vi "Load Data.vi"(5 "LoadData?":bool, 6 "File Info Buffer Input":T1[](array[typedef])=[{"FilePath"=path "/opticsmac/Documents/Optics2mac/DATA/vclong/01:25:02/visibleperp/v14500aEp02.03T", "Field (T)"=2.0, "Temperature (K)"=4.46, "X-Axis"=enum."cm_1", "Center nm"=689.656101368671, "Current Grating Density"=enum."150", "CCD Parameters"={"Exposure Time (s)"=0.2, "Offset"=0.0, "BkgrdCrct"=FALSE, "Shutter"=FALSE, "Mode"=enum."Regular", "Repetition"=4, "dt or s"=0.0}, "Operation Mode"=enum."NML Data Acquisition", "Exp Index"=0, "Index_repetition"=0, "Index"=0, "Current Detector"=enum."CCD-1024x256"}, {"FilePath"=path "", "Field (T)"=0.0, "Temperature (K)"=0.0, "X-Axis"=enum."Point", "Center nm"=0.0, "Current Grating Density"=enum."150", "CCD Parameters"={"Exposure Time (s)"=0.2, "Offset"=0.0, "BkgrdCrct"=FALSE, "Shutter"=FALSE, "Mode"=enum."Regular", "Repetition"=4, "dt or s"=0.0}, "Operation Mode"=enum."Standby", "Exp Index"=0, "Index_repetition"=0, "Index"=0, "Current Detector"=enum."CCD-1024x256"}, {"FilePath"=path "", "Field (T)"=0.0, "Temperature (K)"=0.0, "X-Axis"=enum."Point", "Center nm"=0.0, "Current Grating Density"=enum."150", "CCD Parameters"={"Exposure Time (s)"=0.2, "Offset"=0.0, "BkgrdCrct"=FALSE, "Shutter"=FALSE, "Mode"=enum."Regular", "Repetition"=4, "dt or s"=0.0}, "Operation Mode"=enum."Standby", "Exp Index"=0, "Index_repetition"=0, "Index"=0, "Current Detector"=enum."CCD-1024x256"}, {"FilePath"=path "", "Field (T)"=0.0, "Temperature (K)"=0.0, "X-Axis"=enum."Point", "Center nm"=0.0, "Current Grating Density"=enum."150", "CCD Parameters"={"Exposure Time (s)"=0.2, "Offset"=0.0, "BkgrdCrct"=FALSE, "Shutter"=FALSE, "Mode"=enum."Regular", "Repetition"=4, "dt or s"=0.0}, "Operation Mode"=enum."Standby", "Exp Index"=0, "Index_repetition"=0, "Index"=0, "Current Detector"=enum."CCD-1024x256"}, {"FilePath"=path "", "Field (T)"=0.0, "Temperature (K)"=0.0, "X-Axis"=enum."Point", "Center nm"=0.0, "Current Grating Density"=enum."150", "CCD Parameters"={"Exposure Time (s)"=0.2, "Offset"=0.0, "BkgrdCrct"=FALSE, "Shutter"=FALSE, "Mode"=enum."Regular", "Repetition"=4, "dt or s"=0.0}, "Operation Mode"=enum."Standby", "Exp Index"=0, "Index_repetition"=0, "Index"=0, "Current Detector"=enum."CCD-1024x256"}, {"FilePath"=path "", "Field (T)"=0.0, "Temperature (K)"=0.0, "X-Axis"=enum."Point", "Center nm"=0.0, "Current Grating Density"=enum."150", "CCD Parameters"={"Exposure Time (s)"=0.2, "Offset"=0.0, "BkgrdCrct"=FALSE, "Shutter"=FALSE, "Mode"=enum."Regular", "Repetition"=4, "dt or s"=0.0}, "Operation Mode"=enum."Standby", "Exp Index"=0, "Index_repetition"=0, "Index"=0, "Current Detector"=enum."CCD-1024x256"}, {"FilePath"=path "", "Field (T)"=0.0, "Temperature (K)"=0.0, "X-Axis"=enum."Point", "Center nm"=0.0, "Current Grating Density"=enum."150", "CCD Parameters"={"Exposure Time (s)"=0.2, "Offset"=0.0, "BkgrdCrct"=FALSE, "Shutter"=FALSE, "Mode"=enum."Regular", "Repetition"=4, "dt or s"=0.0}, "Operation Mode"=enum."Standby", "Exp Index"=0, "Index_repetition"=0, "Index"=0, "Current Detector"=enum."CCD-1024x256"}, {"FilePath"=path "", "Field (T)"=0.0, "Temperature (K)"=0.0, "X-Axis"=enum."Point", "Center nm"=0.0, "Current Grating Density"=enum."150", "CCD Parameters"={"Exposure Time (s)"=0.2, "Offset"=0.0, "BkgrdCrct"=FALSE, "Shutter"=FALSE, "Mode"=enum."Regular", "Repetition"=4, "dt or s"=0.0}, "Operation Mode"=enum."Standby", "Exp Index"=0, "Index_repetition"=0, "Index"=0, "Current Detector"=enum."CCD-1024x256"}, {"FilePath"=path "", "Field (T)"=0.0, "Temperature (K)"=0.0, "X-Axis"=enum."Point", "Center nm"=0.0, "Current Grating Density"=enum."150", "CCD Parameters"={"Exposure Time (s)"=0.2, "Offset"=0.0, "BkgrdCrct"=FALSE, "Shutter"=FALSE, "Mode"=enum."Regular", "Repetition"=4, "dt or s"=0.0}, "Operation Mode"=enum."Standby", "Exp Index"=0, "Index_repetition"=0, "Index"=0, "Current Detector"=enum."CCD-1024x256"}, {"FilePath"=path "", "Field (T)"=0.0, "Temperature (K)"=0.0, "X-Axis"=enum."Point", "Center nm"=0.0, "Current Grating Density"=enum."150", "CCD Parameters"={"Exposure Time (s)"=0.2, "Offset"=0.0, "BkgrdCrct"=FALSE, "Shutter"=FALSE, "Mode"=enum."Regular", "Repetition"=4, "dt or s"=0.0}, "Operation Mode"=enum."Standby", "Exp Index"=0, "Index_repetition"=0, "Index"=0, "Current Detector"=enum."CCD-1024x256"}] {"CCD Parameters"."dt or s" format="%#.6f"; "CCD Parameters"."Repetition" min=1; "CCD Parameters"."Offset" format="%#.2f"; "CCD Parameters"."Exposure Time (s)" min=0.02 max=6000.0 format="%#.2f"; "Center nm" format="%.2f"; "Temperature (K)" format="%.2f"; "Field (T)" format="%.2f"}, 7 "Y-Array in":dbl[](array[numeric]), 8 "Y Array Buffer Input":dbl[][](array[numeric])=array1024x10[10240 elements] format="%.2f", 9 "X-Axis Array Input":dbl[][](array[numeric])=array1024x11[11264 elements] format="%.2f") -> (0 "File Info Buffer Out":T1[](array[typedef])=[{"FilePath"=path "/opticsmac/Documents/Optics2mac/DATA/vclong/01:25:02/visibleperp/v14500aEp02.03T", "Field (T)"=2.0, "Temperature (K)"=4.46, "X-Axis"=enum."cm_1", "Center nm"=689.656101368671, "Current Grating Density"=enum."150", "CCD Parameters"={"Exposure Time (s)"=0.2, "Offset"=0.0, "BkgrdCrct"=FALSE, "Shutter"=FALSE, "Mode"=enum."Regular", "Repetition"=4, "dt or s"=0.0}, "Operation Mode"=enum."NML Data Acquisition", "Exp Index"=0, "Index_repetition"=0, "Index"=0, "Current Detector"=enum."CCD-1024x256"}] {"CCD Parameters"."dt or s" format="%#.6f"; "CCD Parameters"."Repetition" min=1; "CCD Parameters"."Offset" format="%#.2f"; "CCD Parameters"."Exposure Time (s)" min=0.02 max=6000.0 format="%#.2f"; "Center nm" format="%.2f"; "Temperature (K)" format="%.2f"; "Field (T)" format="%.2f"}, 1 "Y-Array out":dbl[](array[numeric]), 2 "Data Array output":dbl[][](array[numeric])=[[156320.0], [157260.0], [158740.0], [160150.0], [162530.0], [164140.0], [166060.0], [167590.0], [169200.0], [171260.0], [172690.0], [174810.0], [176260.0], [178620.0], [180480.0], [181740.0], [183460.0], [185700.0], [187270.0], [189260.0], [191040.0], [192940.0], [193980.0], [196750.0], [198840.0], [200170.0], [202190.0], [203860.0], [205040.0], [206430.0], [209340.0], [210440.0], [213240.0], [214740.0], [216720.0], [218710.0], [220610.0], [222540.0], [224090.0], [226040.0], [227760.0], [228770.0], [231810.0], [233660.0], [235500.0], [237390.0], [239590.0], [241700.0], [243190.0], [245260.0], [245670.0], [248540.0], [250180.0], [252160.0], [254040.0], [255810.0], [257360.0], [258980.0], [260540.0], [261970.0], [262240.0], [265810.0], [266800.0], [268760.0], [270660.0], [271180.0], [273130.0], [274420.0], [276410.0], [276090.0], [278520.0], [280230.0], [281030.0], [281870.0], [283440.0], [285750.0], [286320.0], [287530.0], [288750.0], [288670.0], [290950.0], [292320.0], [293710.0], [294870.0], [295370.0], [296240.0], [297700.0], [298710.0], [298800.0], [301150.0], [302130.0], [303180.0], [303690.0], [304680.0], [305540.0], [306660.0], [307720.0], [308220.0], [307800.0], [310510.0], [310980.0], [311540.0], [312460.0], [312990.0], [313790.0], [314260.0], [315080.0], [314160.0], [316990.0], [317280.0], [317390.0], [317810.0], [318990.0], [319270.0], [319920.0], [320880.0], [320580.0], [321670.0], [323440.0], [324260.0], [324090.0], [325340.0], [326440.0], [327880.0], [328190.0], [329450.0], [328800.0], [331840.0], [332880.0], [333390.0], [334690.0], [335400.0], [336540.0], [337530.0], [338800.0], [338680.0], [340000.0], [341080.0], [341600.0], [342840.0], [343390.0], [344390.0], [345420.0], [346090.0], [346340.0], [346460.0], [349550.0], [349420.0], [350670.0], [351070.0], [351930.0], [353120.0], [353520.0], [354520.0], [354640.0], [355380.0], [356380.0], [357290.0], [358190.0], [358930.0], [359670.0], [359540.0], [360830.0], [361900.0], [360600.0], [362480.0], [363660.0], [364070.0], [364740.0], [364990.0], [366060.0], [366930.0], [367780.0], [367940.0], [368640.0], [369950.0], [370430.0], [371320.0], [371730.0], [372740.0], [373400.0], [373890.0], [374850.0], [374640.0], [376240.0], [378000.0], [377860.0], [379380.0], [380050.0], [380630.0], [381640.0], [382180.0], [382230.0], [383250.0], [385270.0], [385380.0], [387220.0], [387590.0], [387980.0], [389810.0], [390380.0], [391030.0], [390020.0], [392370.0], [393610.0], [394220.0], [394720.0], [395770.0], [397090.0], [397800.0], [398480.0], [398130.0], [399860.0], [400870.0], [401860.0], [402070.0], [403020.0], [404320.0], [405070.0], [406210.0], [407160.0], [406140.0], [408920.0], [410760.0], [410970.0], [412260.0], [413420.0], [414890.0], [415800.0], [416960.0], [417480.0], [417970.0], [420910.0], [421760.0], [422450.0], [425020.0], [425520.0], [427330.0], [429060.0], [430200.0], [429790.0], [433380.0], [434550.0], [435800.0], [437460.0], [439590.0], [441200.0], [442140.0], [444010.0], [444080.0], [447490.0], [449670.0], [449930.0], [451710.0], [453330.0], [454340.0], [456010.0], [459020.0], [459170.0], [459650.0], [463490.0], [464920.0], [466220.0], [467140.0], [469790.0], [470470.0], [471550.0], [473460.0], [473170.0], [476510.0], [478130.0], [479950.0], [481700.0], [482610.0], [484720.0], [486310.0], [487360.0], [488710.0], [488480.0], [491530.0], [493680.0], [494030.0], [496330.0], [496710.0], [499040.0], [500660.0], [502060.0], [501750.0], [505120.0], [507080.0], [509080.0], [510410.0], [511400.0], [513950.0], [515830.0], [516880.0], [518020.0], [517880.0], [521810.0], [522630.0], [524040.0], [526020.0], [526400.0], [527650.0], [529510.0], [531110.0], [530100.0], [534120.0], [534870.0], [536820.0], [537820.0], [538610.0], [539780.0], [542010.0], [541950.0], [543990.0], [542980.0], [545900.0], [546330.0], [547660.0], [548080.0], [549810.0], [550340.0], [551570.0], [553330.0], [551440.0], [554700.0], [555680.0], [557650.0], [558440.0], [559220.0], [559960.0], [561330.0], [562400.0], [562300.0], [561740.0], [564550.0], [565120.0], [566410.0], [566540.0], [567600.0], [569260.0], [569370.0], [570620.0], [569700.0], [573110.0], [574280.0], [574450.0], [575220.0], [576960.0], [577570.0], [580100.0], [580380.0], [581520.0], [581380.0], [585270.0], [586540.0], [587260.0], [589060.0], [590240.0], [591500.0], [593040.0], [594340.0], [593420.0], [596370.0], [597700.0], [598570.0], [601150.0], [601800.0], [604910.0], [606790.0], [607480.0], [608140.0], [609520.0], [612450.0], [613670.0], [614660.0], [615130.0], [616330.0], [617050.0], [618050.0], [620390.0], [620190.0], [624180.0], [625540.0], [626790.0], [628820.0], [629000.0], [630620.0], [631500.0], [632660.0], [632820.0], [635130.0], [637650.0], [638560.0], [639160.0], [640430.0], [641030.0], [642840.0], [644020.0], [644840.0], [643680.0], [646820.0], [648710.0], [649660.0], [649440.0], [650920.0], [652720.0], [653450.0], [654620.0], [654780.0], [656430.0], [657460.0], [657570.0], [659320.0], [659400.0], [660680.0], [661770.0], [662130.0], [662360.0], [661080.0], [664420.0], [664320.0], [665300.0], [665760.0], [665580.0], [666220.0], [667220.0], [667340.0], [666260.0], [666190.0], [667200.0], [666770.0], [667620.0], [667530.0], [667110.0], [667250.0], [666860.0], [666590.0], [664350.0], [667200.0], [666880.0], [666520.0], [666110.0], [665080.0], [664700.0], [665990.0], [664640.0], [663420.0], [662240.0], [662810.0], [663050.0], [662600.0], [662030.0], [662160.0], [660780.0], [660130.0], [657870.0], [655800.0], [658220.0], [657800.0], [655630.0], [654120.0], [654570.0], [652660.0], [652060.0], [651740.0], [649510.0], [647850.0], [647320.0], [646010.0], [644610.0], [642420.0], [640220.0], [640340.0], [638990.0], [637100.0], [633820.0], [634320.0], [632920.0], [631980.0], [630800.0], [629090.0], [628850.0], [627160.0], [625590.0], [623130.0], [621440.0], [621550.0], [620700.0], [618500.0], [617880.0], [616220.0], [615470.0], [612630.0], [611170.0], [607430.0], [608600.0], [606890.0], [604420.0], [603270.0], [601590.0], [599460.0], [597450.0], [596090.0], [592650.0], [591760.0], [591090.0], [589220.0], [586320.0], [586060.0], [584040.0], [581410.0], [580850.0], [578450.0], [574310.0], [574760.0], [572940.0], [570980.0], [569590.0], [567810.0], [565600.0], [563760.0], [561900.0], [557600.0], [557220.0], [554640.0], [552400.0], [551480.0], [549700.0], [548050.0], [546890.0], [545140.0], [542510.0], [538000.0], [538080.0], [536770.0], [534010.0], [531830.0], [530640.0], [529320.0], [527240.0], [525000.0], [520960.0], [521070.0], [520170.0], [518210.0], [516210.0], [515020.0], [512950.0], [511720.0], [510620.0], [508390.0], [503950.0], [504510.0], [503570.0], [501270.0], [500230.0], [498290.0], [497320.0], [496810.0], [493930.0], [490820.0], [491560.0], [489960.0], [489310.0], [486820.0], [485200.0], [484360.0], [481680.0], [480350.0], [478600.0], [474800.0], [474770.0], [472460.0], [471520.0], [469300.0], [467320.0], [465240.0], [463430.0], [461630.0], [456970.0], [457570.0], [455660.0], [453120.0], [450930.0], [448980.0], [446190.0], [444850.0], [443350.0], [441040.0], [436880.0], [436140.0], [434420.0], [432330.0], [430310.0], [428480.0], [426040.0], [424900.0], [422610.0], [419380.0], [418430.0], [416630.0], [416290.0], [414300.0], [412500.0], [411400.0], [410060.0], [408660.0], [407070.0], [403290.0], [403090.0], [401900.0], [400240.0], [399050.0], [397450.0], [395580.0], [394440.0], [393710.0], [390260.0], [390640.0], [388280.0], [386530.0], [385640.0], [384440.0], [382570.0], [381800.0], [381000.0], [378720.0], [377390.0], [376850.0], [375200.0], [374320.0], [373100.0], [371220.0], [370010.0], [368870.0], [367560.0], [364680.0], [364510.0], [363130.0], [361300.0], [360060.0], [358740.0], [357360.0], [355990.0], [354730.0], [352870.0], [351670.0], [351570.0], [350560.0], [349430.0], [349280.0], [348110.0], [348810.0], [348240.0], [347840.0], [346100.0], [347600.0], [347650.0], [348340.0], [348530.0], [348790.0], [348900.0], [348490.0], [349230.0], [348620.0], [347720.0], [349040.0], [348820.0], [348160.0], [348370.0], [348810.0], [348410.0], [348440.0], [348090.0], [346440.0], [347530.0], [347510.0], [347190.0], [346980.0], [346970.0], [347380.0], [346650.0], [346660.0], [346160.0], [345540.0], [346110.0], [346250.0], [346100.0], [346130.0], [345360.0], [345870.0], [346100.0], [345550.0], [344440.0], [345530.0], [345280.0], [345730.0], [345620.0], [345010.0], [345010.0], [345170.0], [345320.0], [343740.0], [344220.0], [345060.0], [344330.0], [345130.0], [344780.0], [344760.0], [344580.0], [344900.0], [344560.0], [343020.0], [343620.0], [343590.0], [343780.0], [342910.0], [343500.0], [343130.0], [343920.0], [343120.0], [342650.0], [342610.0], [343040.0], [343040.0], [342780.0], [342740.0], [342160.0], [341750.0], [341210.0], [340920.0], [339020.0], [340380.0], [339050.0], [338350.0], [337570.0], [337100.0], [336350.0], [335800.0], [335510.0], [333940.0], [333380.0], [334120.0], [334050.0], [333630.0], [334510.0], [334900.0], [335700.0], [337260.0], [338810.0], [339090.0], [343020.0], [345650.0], [347530.0], [350990.0], [354050.0], [357380.0], [360650.0], [363900.0], [365580.0], [369540.0], [373470.0], [375250.0], [377750.0], [379810.0], [381750.0], [383410.0], [384500.0], [386600.0], [385600.0], [387930.0], [389910.0], [390520.0], [391700.0], [392050.0], [391960.0], [391730.0], [392450.0], [390690.0], [393050.0], [392850.0], [393580.0], [394080.0], [392820.0], [393180.0], [392870.0], [392970.0], [393260.0], [390860.0], [391510.0], [391330.0], [390430.0], [389300.0], [388920.0], [388670.0], [388150.0], [388100.0], [386960.0], [388040.0], [388650.0], [387730.0], [387970.0], [386880.0], [387000.0], [386420.0], [386990.0], [385910.0], [383510.0], [384780.0], [384030.0], [384080.0], [383180.0], [381830.0], [381580.0], [381410.0], [381920.0], [379820.0], [381400.0], [381260.0], [381480.0], [381220.0], [381160.0], [380220.0], [379490.0], [379530.0], [379140.0], [377530.0], [378270.0], [377830.0], [377610.0], [376940.0], [376510.0], [376080.0], [375890.0], [376230.0], [373670.0], [374800.0], [374290.0], [373960.0], [373110.0], [373330.0], [372760.0], [371680.0], [371860.0], [371300.0], [367850.0], [368940.0], [368290.0], [367740.0], [367630.0], [366490.0], [366590.0], [365400.0], [364700.0], [362360.0], [362780.0], [362460.0], [361600.0], [361410.0], [360710.0], [359930.0], [359220.0], [358090.0], [358030.0], [355680.0], [356970.0], [355700.0], [355970.0], [355130.0], [354980.0], [354470.0], [354120.0], [353610.0], [351920.0], [353430.0], [353730.0], [353240.0], [352810.0], [352730.0], [352930.0], [353230.0], [352990.0], [352320.0], [352370.0], [353100.0], [353530.0], [354110.0], [353310.0], [354720.0], [354820.0], [355090.0], [356000.0], [354730.0], [356760.0], [357560.0], [358070.0], [358370.0], [359300.0], [359980.0], [361140.0], [362240.0], [362300.0], [362850.0], [364220.0], [365530.0], [366740.0], [367400.0], [368790.0], [369320.0], [370690.0], [372240.0], [370660.0], [374080.0], [374970.0], [376000.0], [377270.0], [378520.0], [379880.0], [381660.0], [383190.0], [384070.0], [384140.0], [386260.0], [388280.0], [389600.0], [391170.0], [392920.0], [393800.0], [395680.0], [397070.0], [397120.0], [400470.0], [401730.0], [403790.0], [406060.0], [406910.0], [408630.0], [411080.0], [413560.0], [413080.0], [415620.0], [418270.0], [419420.0], [421620.0], [423980.0], [426180.0], [427900.0], [429930.0], [431090.0], [432040.0], [435340.0], [437000.0], [439230.0], [441180.0], [442820.0], [445160.0], [447410.0], [448810.0], [450420.0], [452100.0], [453960.0], [456590.0], [457360.0], [460200.0], [462210.0], [464290.0], [466050.0], [467300.0], [467040.0], [470870.0], [472490.0], [475020.0], [476600.0], [479850.0], [481770.0], [483830.0], [485770.0], [487240.0], [489490.0], [491690.0], [493030.0], [495820.0], [497760.0], [499750.0], [502150.0], [504600.0], [507830.0], [505690.0], [510100.0], [512330.0], [514740.0], [516420.0], [517990.0], [520020.0], [521630.0], [523580.0], [524160.0], [525290.0], [528610.0], [529240.0], [531820.0], [533720.0], [536570.0], [537640.0], [539530.0], [541010.0], [542030.0], [545080.0], [547040.0], [548830.0], [550910.0], [551940.0], [553730.0], [556100.0], [556780.0], [557540.0], [560360.0], [562490.0], [563420.0], [565890.0], [565840.0], [556840.0]] format="%.2f", 3 "X-Axis Array output":dbl[][](array[numeric])=[[569.9785612360697], [570.2125422703458], [570.4467790424538], [570.6811447284165], [570.9150664597546], [571.149498604365], [571.3834857004028], [571.6176645935107], [571.8520993896819], [572.0859594909508], [572.3203947937624], [572.5543820427264], [572.7885606964572], [573.0228668580249], [573.257108052247], [573.4911554110627], [573.7251368031901], [573.959566566362], [574.1935440459157], [574.4277123674399], [574.6618137673706], [574.8960415039011], [575.1301372348125], [575.3644236893715], [575.598512842311], [575.8325335034439], [576.0667445331885], [576.3007569575373], [576.5350245027386], [576.7690927467231], [577.0034161532332], [577.237539561065], [577.4715925143892], [577.7057701635956], [577.9398116322578], [578.1740428085933], [578.4081372083515], [578.6424212478402], [578.8765679131884], [579.1105766403081], [579.3447090835253], [579.5787684902041], [579.8130170966701], [580.047060849429], [580.281030556443], [580.5151232693252], [580.7494049303583], [580.9836120636254], [581.2176123012891], [581.4518011094145], [581.6858482876963], [581.9197532660246], [582.1541773939755], [582.3881280180103], [582.6222667533773], [582.8561957158248], [583.0903790087464], [583.3244182677612], [583.5585789664744], [583.7926614753968], [584.0268652358009], [584.2609236252295], [584.4949027934747], [584.7290026613164], [584.9632901260253], [585.1970965537491], [585.4314246553758], [585.6652705642005], [585.8996385960471], [586.1334561771368], [586.3675276076606], [586.6017860649538], [586.8358954680223], [587.0697879210392], [587.3038668912492], [587.5378629136461], [587.771977993909], [588.0059420756725], [588.2401600748535], [588.4741589158375], [588.708343997923], [588.9423768195961], [589.1762567952333], [589.4103226008467], [589.644574458002], [589.8786048264974], [590.1125489853926], [590.3466787810725], [590.580585701375], [590.8147462283345], [591.0486831331444], [591.2828053689865], [591.5168398027985], [591.7509911829102], [591.9849857807982], [592.2188230044163], [592.4528450349327], [592.6870520915197], [592.9211010776456], [593.1549913992526], [593.3890663196886], [593.6229131024171], [593.8570131497573], [594.0912979084737], [594.3250087204426], [594.5593177431829], [594.7930515160485], [595.0273840434575], [595.2611400157674], [595.4950797219038], [595.7292033785758], [595.9631643548844], [596.1973091705743], [596.4312906493552], [596.6651081898347], [596.8991091280797], [597.1332936799505], [597.367313577354], [597.6010984655192], [597.8351362188375], [598.0692874950604], [598.3033425992447], [598.5371611499348], [598.7712325507011], [599.0050666235196], [599.2390834029617], [599.4732831032484], [599.7069634997492], [599.9411776423483], [600.1752230319117], [600.4090990591753], [600.6431574309179], [600.877045769227], [601.1111163290896], [601.3449455547924], [601.5790274511555], [601.8128672292677], [602.0469596628537], [602.2808091924991], [602.514911361466], [602.748769839205], [602.9828099258036], [603.216747558975], [603.450795659303], [603.6846695575144], [603.918368637198], [604.1526051721127], [604.386238691957], [604.6204813770987], [604.8541911551888], [605.0880816793274], [605.3220815938698], [605.5559760805389], [605.7900513892174], [606.0238773407672], [606.2578838686974], [606.4917838131607], [606.7257924111401], [606.9596218926068], [607.1936316772918], [607.4275337172702], [607.661543913694], [607.89537360751], [608.1293833271114], [608.3631395625441], [608.597147914069], [608.8309743709509], [609.0649805717787], [609.2987316709077], [609.5327348245695], [609.766845166383], [610.0004813285047], [610.234587524326], [610.4685459360591], [610.7023195953143], [610.9362359168458], [611.1700032032709], [611.4039129492185], [611.6380018097078], [611.871904377806], [612.1056200202532], [612.339514274836], [612.5735507012292], [612.8074360352316], [613.0410963234237], [613.2749348664887], [613.5089886256392], [613.7428164669835], [613.976822614781], [614.2106388600395], [614.4445963888058], [614.6784001409918], [614.9123449658256], [615.1461353534156], [615.3800666016712], [615.6138057407791], [615.84772250912], [616.0814464485342], [616.3153478591558], [616.5494269431979], [616.783275246885], [617.0169663999313], [617.2507974982777], [617.4848058938925], [617.718656418489], [617.9522366370846], [618.1860308913114], [618.4200021185717], [618.6537767574555], [618.887728205784], [619.1214449036934], [619.3553381897889], [619.5890333709201], [619.8229424919921], [620.0569907459521], [620.2908400791476], [620.5244522387055], [620.7582780601838], [620.9922801684296], [621.2260441981704], [621.4600220047827], [621.6937609388353], [621.927675763351], [622.1613886642195], [622.3952772840859], [622.6289632400833], [622.8627868559894], [623.0964449244505], [623.3302404222478], [623.564249405239], [623.7980161517389], [624.0315779479429], [624.2656952832338], [624.4992266333307], [624.7333139161664], [624.9668138959906], [625.2008320299667], [625.4346816845912], [625.6682858277579], [625.9020645416273], [626.1360563077307], [626.3698016352901], [626.6033381191387], [626.8374325277452], [627.0708955086782], [627.3049551761817], [627.5383820307816], [627.7724060186698], [628.0061809545841], [628.2397446303601], [628.4734821015171], [628.7073935621099], [628.9410929104458], [629.174966062032], [629.4086263402593], [629.6424215186693], [629.8760417482332], [630.1097966320631], [630.3437250790315], [630.5774389737746], [630.8113651016672], [631.0449981919082], [631.2788433245437], [631.5124723713293], [631.7462744089887], [631.979820588088], [632.2135395073883], [632.4474704201107], [632.6811445201904], [632.9149913579909], [633.1486196432628], [633.3824204709198], [633.6160019721298], [633.8497165843745], [634.083642939327], [634.3173098008219], [634.5507950475294], [634.7848064008625], [635.0182028215893], [635.2521650218868], [635.4859053073872], [635.7194229977089], [635.9531123694371], [636.1869340871817], [636.4205718226408], [636.6543416437656], [636.8879267568933], [637.1216436942005], [637.3555322273472], [637.5891955529648], [637.8226329866419], [638.0566389917908], [638.2899812471152], [638.5239322074651], [638.7576562808872], [638.9911129066096], [639.2247402447219], [639.4585384825399], [639.692148153701], [639.9258885830285], [640.1597998900476], [640.3934417207572], [640.626893454426], [640.8605154571301], [641.0942677783141], [641.3277890211948], [641.5615206436516], [641.7953824702491], [642.0290123129754], [642.2628123120527], [642.496379526627], [642.7301166825058], [642.9635798805645], [643.1972531457308], [643.4310963211325], [643.6646645385084], [643.8984023899698], [644.1319453967337], [644.3656173302636], [644.5990530940628], [644.8326174473822], [645.066391757513], [645.2999289791973], [645.5336353598614], [645.7674703591786], [646.0011080433068], [646.2344662336811], [646.4684012053606], [646.7016887629393], [646.9355534678967], [647.1691783656399], [647.4025627531603], [647.6361155291756], [647.8697958862166], [648.103685956802], [648.3372934247961], [648.5706996532427], [648.8042328900535], [649.0379343657853], [649.2713925888587], [649.5050188216914], [649.7388132457125], [649.9723634797793], [650.2060403887166], [650.4395135398449], [650.6731130749776], [650.9069218357406], [651.140443235878], [651.3737179101438], [651.6075744289843], [651.8411839880306], [652.074545875291], [652.308074911467], [652.5417296931276], [652.7755935365271], [653.0087505723392], [653.242532621299], [653.476023396739], [653.7097228787869], [653.9431301933079], [654.1767042437094], [654.4104452087186], [654.643892901282], [654.8775490900751], [655.1109530200998], [655.3444814426795], [655.5782183880856], [655.8116601135669], [656.0453101793759], [656.2786641242704], [656.5121841352549], [656.7458703896632], [656.9793015591454], [657.2128987273431], [657.4466198608332], [657.6801271223752], [657.913335337913], [658.147174305523], [658.3807139200136], [658.613995727499], [658.8474853001089], [659.0810980625783], [659.3148765516596], [659.5483961348145], [659.7816135745428], [660.0154639560657], [660.2486287429053], [660.4823417401426], [660.7158365714216], [660.9494538905137], [661.182809556881], [661.4163300591503], [661.6500155720365], [661.883438448266], [662.1170260806862], [662.3503502177476], [662.5838388554693], [662.8174492648519], [663.0508380632363], [663.2843483160027], [663.5175931625031], [663.7514753723896], [663.9846183813248], [664.2183560764337], [664.4518272425249], [664.6850311438042], [664.9188305532281], [665.1523192315412], [665.3855828228633], [665.6189668124593], [665.852557875202], [666.085836348174], [666.3192783345766], [666.5529273943554], [666.7862627704383], [667.0197615677935], [667.2534239581643], [667.4867715072842], [667.7203258631687], [667.9536080127298], [668.1870096223497], [668.4206180344975], [668.6539095684766], [668.8873640056947], [669.1209815168397], [669.3543684916073], [669.5878745482652], [669.8210616205942], [670.0544550114707], [670.2880111068818], [670.5217300770249], [670.7551287876049], [670.9882943339953], [671.2215780432409], [671.4550240212379], [671.6886764964981], [671.9220066530777], [672.1554989737157], [672.3887121169042], [672.62204296728], [672.8555800261507], [673.0892793113455], [673.3226982539178], [673.555791797064], [673.7895344693354], [674.0225077441829], [674.2560861488573], [674.4893822263485], [674.7228398030073], [674.9565035354801], [675.1897949282433], [675.4228466922716], [675.6565052063161], [675.8898793213142], [676.1233700656283], [676.3566201244364], [676.5899864682003], [676.8235139064099], [677.0567997098706], [677.2902015884175], [677.5233161643367], [677.7570398537687], [677.9899821683338], [678.2235787871269], [678.4568869138255], [678.6903556112117], [678.923489897466], [679.1568294491952], [679.3902843739306], [679.6239449568319], [679.8572698087271], [680.0903032405772], [680.3239484726362], [680.5573019943785], [680.7903630401039], [681.0235384746044], [681.2569190155838], [681.4904595661528], [681.7236610504576], [681.9570676059204], [682.1905885945728], [682.4238147784475], [682.6572459966719], [682.8903360147227], [683.1235852620623], [683.3569939019063], [683.5905620976938], [683.8237876919464], [684.0572181797826], [684.2903508110712], [684.5235966447381], [684.7570473302867], [684.9901532665468], [685.2234179653401], [685.4568874728135], [685.6900110634476], [685.9232932784943], [686.1567342799079], [686.3898281317407], [686.623126445873], [686.856583406323], [687.0897381470143], [687.3230050969968], [687.5564766544361], [687.789598713726], [688.0228789107953], [688.2563636660593], [688.4894977448944], [688.7227898169376], [688.9562400428498], [689.1893847335801], [689.4226872713384], [689.656101368671], [689.8892552578118], [690.1225668461884], [690.3555243307512], [690.5891514513938], [690.8224240958862], [691.055388021864], [691.2885091242657], [691.5217875622108], [691.7552234950339], [691.9883494570898], [692.2216326020165], [692.4550730888359], [692.6882025052314], [692.9214420615496], [693.154885662274], [693.3879701385429], [693.621258407787], [693.854186542698], [694.0877416377679], [694.3210303127407], [694.5539105419989], [694.7875127414463], [695.0202343195562], [695.2536311046698], [695.4867123324328], [695.7199498918577], [695.9532966403738], [696.1863739873769], [696.4195601403177], [696.6529499510642], [696.8859745504592], [697.119155091584], [697.352491731027], [697.5855094050058], [697.8191583932959], [698.052012237179], [698.2854977081029], [698.5186629315928], [698.7514594284022], [698.9849359872462], [699.2180434308635], [699.4513541829035], [699.6842947933923], [699.9173906095419], [700.1506896586855], [700.3840963837952], [700.6171794206019], [700.8504176459352], [701.0833312166185], [701.316351615363], [701.5495750281236], [701.7829536098167], [702.0159581115853], [702.2491655476285], [702.4824797851062], [702.7155150939038], [702.9486568085897], [703.1819532746579], [703.4149214500542], [703.6480440439698], [703.8813212099857], [704.1142689444213], [704.347370916823], [704.5806272804261], [704.8140381886692], [705.0470698099189], [705.2803041521312], [705.5131581648886], [705.7461659857089], [705.9793764395791], [706.2126923662339], [706.4456751899384], [706.6788117885895], [706.9121023144813], [707.145058585656], [707.3781684445645], [707.6114320431471], [707.844311302739], [708.0773928590395], [708.3106279657914], [708.5434774801842], [708.7764801384772], [709.0096851830824], [709.2429946150864], [709.4759660859403], [709.7090906595838], [709.9423684869894], [710.1753071906984], [710.4083988032949], [710.6416434753902], [710.8745478587958], [711.1075555733332], [711.3407655013067], [711.5735845262209], [711.806605481884], [712.039729591787], [712.273055997113], [712.5059900253336], [712.7390764558131], [712.9723154381692], [713.2052103819556], [713.4382575273833], [713.6714570237015], [713.9042615343643], [714.1372677833431], [714.3704261805599], [714.6031883165729], [714.8366510991905], [715.0697172024965], [715.3024856342254], [715.5353556570582], [715.7683773530886], [716.0015508705467], [716.2348763578561], [716.4678526681815], [716.70047897149], [716.9337583312919], [717.1666873272304], [717.3997174678144], [717.6329493880252], [717.8658297547535], [718.0988109574024], [718.3319938265538], [718.5647735268387], [718.7977041432862], [719.0307858227071], [719.2640692336621], [719.4969479698311], [719.7299775548271], [719.9626013176862], [720.1959326794039], [720.4289084763316], [720.6620350524665], [720.8947542938646], [721.1276746688834], [721.3606947886973], [721.5939163995395], [721.8267291591917], [722.0597431103231], [722.2928566012382], [722.5256108516573], [722.758515157566], [722.991569664121], [723.2242637220327], [723.457618736422], [723.6906129341463], [723.9231942941278], [724.1564885199274], [724.3893694728172], [724.6224515350356], [724.8551192291109], [725.0879877278858], [725.3209545223762], [725.5540710668876], [725.7868230850675], [726.0197244811866], [726.2528269072134], [726.48602752403], [726.7188106338266], [726.9517945770532], [727.1844115522902], [727.4176941796782], [727.6505577576538], [727.8831048166599], [728.1162665155825], [728.349111385633], [728.5820533875615], [728.8151444370693], [729.0479175287326], [729.2807874181402], [729.5138061200224], [729.7464537279817], [729.979249769529], [730.2121423154941], [730.4452356174513], [730.677956402216], [730.9108255245195], [731.1437909220073], [731.3769571118838], [731.6096970864359], [731.8426375379956], [732.0756740332973], [732.3083352779314], [732.5411444538945], [732.7741541396158], [733.00725963518], [733.2399884457418], [733.4728650854023], [733.705837124326], [733.9384837705344], [734.1712780007656], [734.4041672846467], [734.6372570710988], [734.8699674863099], [735.1027726080894], [735.335725280871], [735.5683501029508], [735.8010692827844], [736.0339357646509], [736.266949688449], [736.4995814754819], [736.7323603142135], [736.9652863441196], [737.1983597048528], [737.4310494767265], [737.6638861876831], [737.8968168039282], [738.1294157114595], [738.3626404655607], [738.5950004475568], [738.827986486663], [739.0605861515492], [739.2939194374667], [739.5262785318844], [739.759318149966], [739.9919699308888], [740.2247680942306], [740.4577127781887], [740.6902683570029], [740.923506160012], [741.1563544603426], [741.3887587074263], [741.6218995732415], [741.8545959196258], [742.0874921153204], [742.319942649985], [742.5525927014187], [742.7858735473785], [743.0182227395939], [743.251256813197], [743.4838972932176], [743.7166834535531], [743.949669480017], [744.1821525352484], [744.4148350535932], [744.6476631225607], [744.8806368787639], [745.1131600591114], [745.3458827064325], [745.5786964867079], [745.8117100741464], [746.044271461905], [746.2770323186055], [746.5098840387293], [746.7423365567711], [746.9754787791853], [747.2082213919584], [747.4405635117911], [747.6735960821903], [747.9062277508853], [748.1390042269853], [748.3713787120207], [748.6043901407339], [748.8370538614945], [749.0698622494173], [749.3027606099149], [749.5353100668009], [749.7679490163653], [750.0007324225902], [750.233110761735], [750.4662381436045], [750.6989050792552], [750.9317163270375], [751.1641209978687], [751.3966695663436], [751.6293621661489], [751.8621989311368], [752.0951247563495], [752.3276974878573], [752.5604141022473], [752.7932193915123], [753.0256703803677], [753.2582095581994], [753.4909478437834], [753.7237745161723], [753.9561899913641], [754.1887488443199], [754.4214512077558], [754.6543528300939], [754.886786149125], [755.1199195325336], [755.352026869878], [755.5848902206728], [755.8173393207254], [756.0504897014332], [756.282610994813], [756.5154896546507], [756.7478966066582], [756.9810619453718], [757.2131951498128], [757.4460870734576], [757.678505615293], [757.9116278002577], [758.1437708605221], [758.376673992457], [758.6091020646318], [758.8416164156413], [759.0743296109781], [759.3071855819429], [759.5396210802211], [759.7721989261688], [760.0049192505907], [760.2377257429041], [760.470166621687], [760.7026931698258], [760.9354185044483], [761.1682297003532], [761.4006172549887], [761.6332033995022], [761.8658750007254], [762.0981216216317], [762.331077409063], [762.5636077837489], [762.7962800570787], [763.028525791631], [763.2614819049635], [763.494011045611], [763.7266249495914], [763.9588676786684], [764.1918219982317], [764.4242907165299], [764.6569580124176], [764.8891385070066], [765.1220889028531], [765.354551991043], [765.5871563782794], [765.8193294593644], [766.0522164830647], [766.2846717622601], [766.5173255372134], [766.7494316769349], [766.9823103469583], [767.2147556975435], [767.4473419828546], [767.6800693311062], [767.9123044148358], [768.1447376721959], [768.3772540222936], [768.6099688712962], [768.8421897346353], [769.0751863373794], [769.3076884415051], [769.5397528529897], [769.7725938404661], [770.0049388598031], [770.237424181634], [770.4700499330804], [770.7028162414178], [770.935142822511], [771.1676095144611], [771.4001583328958], [771.6323241301861], [771.8652115298873], [772.0975991685474], [772.3301850319092], [772.5622699146975], [772.7951358583659], [773.0275003023413], [773.260062914976], [773.4921228060754], [773.7249066429874], [773.9572456645357], [774.1897242644668], [774.4224011359809], [774.6545146774336], [774.887471053337], [775.1198635062366], [775.3518670192801], [775.5845968899058], [775.8168787295938], [776.0492409306255], [776.2818012103022], [776.5145009153999], [776.7466920565741], [776.9790220975414], [777.2115501529908], [777.4441584030325], [777.6763153210132], [777.9092609869617], [778.1416958032858], [778.3736778954418], [778.6063903663274], [778.8386496550254], [779.07104755156], [779.303584180046], [779.5356068875016], [779.7684209628557], [780.00078000078], [780.2332775588451], [780.4652594258139], [780.698034005651], [780.9302923623035], [781.1627485455421], [781.3952835316442], [781.6273603772329], [781.8602317940714], [782.0925849450691], [782.3244785509395], [782.5571077545219], [782.7892769488586], [783.0215839440813], [783.254028862911], [783.4866118282148], [783.718733143159], [783.9515922141052], [784.1839291152866], [784.4158629723539], [784.6485353086861], [784.8806839560654], [785.1130302081439], [785.3454538315042], [785.578015108261], [785.8101714378415], [786.0424046848741], [786.2747752379038], [786.507283218738], [786.7393242969458], [786.9721676226125], [787.2044831295315], [787.436269760594], [787.6688593962626], [787.9009802365349], [788.1332379261105], [788.3656325860463], [788.5981036063885], [788.8307725349462], [789.0629707696862], [789.2952449046714], [789.5277167020348], [789.7596554673503], [789.9917305455472], [790.2246128574637], [790.4563511392375], [790.6888359137664], [790.921457482874], [791.1536658383246], [791.3859494216275], [791.6183694424177], [791.8502524563984], [792.0829453171151], [792.3151619255425], [792.5475147327539], [792.7793900894214], [793.0119538807791], [793.2441011184819], [793.4763843140877], [793.7087420662068], [793.9406203746562], [794.1733117283034], [794.4054615996114], [794.637808897988], [794.8696134387612], [795.1021706289258], [795.334246207211], [795.5664573021658], [795.7988040325239], [796.0312865171579], [796.263285699578], [796.4954201513341], [796.7276899907661], [796.9600953363514], [797.1926363067062], [797.4246299392921], [797.656820772043], [797.8890846903162], [798.1209240494411], [798.3534583634893], [798.5855677027041], [798.817749730399], [799.0500668072964], [799.2825814392066], [799.5145447623521], [799.746642762781], [799.9788755578173], [800.2112432649212], [800.4431203086334], [800.675757829049], [800.9079041945205], [801.1395584328427], [801.3719738621262], [801.6044614298306], [801.8365188455465], [802.0687106573157], [802.3009741218762], [802.5328060755495], [802.7653384428093], [802.9974388773092], [803.2296105575747], [803.461286112407], [803.6937892129381], [803.9257326499442], [804.1578100018542], [804.3900213846773], [804.6223669145569], [804.8542140995525], [805.0868912041427], [805.3189428710359], [805.5511917162275], [805.7829404892315], [806.0154570780633], [806.2474730952305], [806.4795592085159], [806.7118425298484], [806.9435602081946], [807.1761109293301], [807.408159095993], [807.640277020615], [807.8725284445685], [808.1043395281949], [808.3362198725039], [808.5688717882188]] format="%.2f", 4 "Dataload Type":u8(ring) items=["None", "Buffer", "File"])   [LabVIEW 2020]
doc: "This is a sub VI to load data into PlotBuffer.\nIt uses the x-arrayPlotBuffer (nm), data-arrayPlotBuffer and FileInfoBuffer as input and output. \nIt should be used in a shift-register settings"
uses:
  Globals and TypeDefs/Type Definitions.llb/FileInfoParameter.ctt
  Globals and TypeDefs/Type Definitions.llb/Wavelength Unit.ctt
  Globals and TypeDefs/Type Definitions.llb/McPherson Grating Density.ctl
  Globals and TypeDefs/Type Definitions.llb/CCDParameter.ctt
  Globals and TypeDefs/Type Definitions.llb/OperationMode.ctt
  Globals and TypeDefs/Type Definitions.llb/ListOfDetectors.ctt
  Globals and TypeDefs/Type Definitions.llb/3 way Status.ctl
  File and save/X-Axis Converter.llb/X-Axis Converter.vi
  File and save/X-Axis_Generator_morph.vi
panel:
  out "File Contents":string="#   FILE:   v14500aEp02.03T\r#   Sample:   NENB #3(transmittance)\r#   Friday, January 25, 2002 9:15 PM\r#   Magnet ID: Cell 8\r#   Magnetic Field (Tesla):      2.03\r#   Temperature (K):     -1.00\r#   Exposure Time:      3.00\r#   User Name:   VCLong\r#   Voigt probe\r#   sample axis parallel to field\r#   100 um slit\r#   no filter  in collection\r#   900nm short pass filter in front of source\r#   visible polarizer perpendicular to sample axis\r#   150 line grating\r#   T=4.5K\r#   Unit\r#   cm_1            Response\r17544.52\t 1.5632E+5\r17537.32\t 1.5726E+5\r17530.12\t 1.5874E+5\r17522.92\t 1.6015E+5\r17515.74\t 1.6253E+5\r17508.55\t 1.6414E+5\r17501.38\t 1.6606E+5\r17494.21\t 1.6759E+5\r17487.04\t 1.6920E+5\r17479.89\t 1.7126E+5\r17472.73\t 1.7269E+5\r17465.59\t 1.7481E+5\r17458.45\t 1.7626E+5\r17451.31\t 1.7862E+5\r17444.18\t 1.8048E+5\r17437.06\t 1.8174E+5\r17429.95\t 1.8346E+5\r17422.83\t 1.8570E+5\r17415.73\t 1.8727E+5\r17408.63\t 1.8926E+5\r17401.54\t 1.9104E+5\r17394.45\t 1.9294E+5\r17387.37\t 1.9398E+5\r17380.29\t 1.9675E+5\r17373.22\t 1.9884E+5\r17366.16\t 2.0017E+5\r17359.10\t 2.0219E+5\r17352.05\t 2.0386E+5\r17345.00\t 2.0504E+5\r17337.96\t 2.0643E+5\r17330.92\t 2.0934E+5\r17323.89\t 2.1044E+5\r17316.87\t 2.1324E+5\r17309.85\t 2.1474E+5\r17302.84\t 2.1672E+5\r17295.83\t 2.1871E+5\r17288.83\t 2.2061E+5\r17281.83\t 2.2254E+5\r17274.84\t 2.2409E+5\r17267.86\t 2.2604E+5\r17260.88\t 2.2776E+5\r17253.91\t 2.2877E+5\r17246.94\t 2.3181E+5\r17239.98\t 2.3366E+5\r17233.03\t 2.3550E+5\r17226.08\t 2.3739E+5\r17219.13\t 2.3959E+5\r17212.19\t 2.4170E+5\r17205.26\t 2.4319E+5\r17198.33\t 2.4526E+5\r17191.41\t 2.4567E+5\r17184.50\t 2.4854E+5\r17177.58\t 2.5018E+5\r17170.68\t 2.5216E+5\r17163.78\t 2.5404E+5\r17156.89\t 2.5581E+5\r17150.00\t 2.5736E+5\r17143.12\t 2.5898E+5\r17136.24\t 2.6054E+5\r17129.37\t 2.6197E+5\r17122.50\t 2.6224E+5\r17115.64\t 2.6581E+5\r17108.79\t 2.6680E+5\r17101.94\t 2.6876E+5\r17095.09\t 2.7066E+5\r17088.26\t 2.7118E+5\r17081.42\t 2.7313E+5\r17074.60\t 2.7442E+5\r17067.77\t 2.7641E+5\r17060.96\t 2.7609E+5\r17054.15\t 2.7852E+5\r17047.34\t 2.8023E+5\r17040.54\t 2.8103E+5\r17033.75\t 2.8187E+5\r17026.96\t 2.8344E+5\r17020.18\t 2.8575E+5\r17013.40\t 2.8632E+5\r17006.63\t 2.8753E+5\r16999.86\t 2.8875E+5\r16993.10\t 2.8867E+5\r16986.34\t 2.9095E+5\r16979.59\t 2.9232E+5\r16972.85\t 2.9371E+5\r16966.11\t 2.9487E+5\r16959.37\t 2.9537E+5\r16952.64\t 2.9624E+5\r16945.92\t 2.9770E+5\r16939.20\t 2.9871E+5\r16932.49\t 2.9880E+5\r16925.78\t 3.0115E+5\r16919.08\t 3.0213E+5\r16912.38\t 3.0318E+5\r16905.69\t 3.0369E+5\r16899.00\t 3.0468E+5\r16892.32\t 3.0554E+5\r16885.65\t 3.0666E+5\r16878.98\t 3.0772E+5\r16872.31\t 3.0822E+5\r16865.65\t 3.0780E+5\r16859.00\t 3.1051E+5\r16852.35\t 3.1098E+5\r16845.71\t 3.1154E+5\r16839.07\t 3.1246E+5\r16832.43\t 3.1299E+5\r16825.81\t 3.1379E+5\r16819.18\t 3.1426E+5\r16812.57\t 3.1508E+5\r16805.95\t 3.1416E+5\r16799.35\t 3.1699E+5\r16792.75\t 3.1728E+5\r16786.15\t 3.1739E+5\r16779.56\t 3.1781E+5\r16772.97\t 3.1899E+5\r16766.39\t 3.1927E+5\r16759.82\t 3.1992E+5\r16753.25\t 3.2088E+5\r16746.68\t 3.2058E+5\r16740.12\t 3.2167E+5\r16733.57\t 3.2344E+5\r16727.02\t 3.2426E+5\r16720.47\t 3.2409E+5\r16713.93\t 3.2534E+5\r16707.40\t 3.2644E+5\r16700.87\t 3.2788E+5\r16694.35\t 3.2819E+5\r16687.83\t 3.2945E+5\r16681.31\t 3.2880E+5\r16674.81\t 3.3184E+5\r16668.30\t 3.3288E+5\r16661.80\t 3.3339E+5\r16655.31\t 3.3469E+5\r16648.82\t 3.3540E+5\r16642.34\t 3.3654E+5\r16635.86\t 3.3753E+5\r16629.39\t 3.3880E+5\r16622.92\t 3.3868E+5\r16616.46\t 3.4000E+5\r16610.00\t 3.4108E+5\r16603.55\t 3.4160E+5\r16597.10\t 3.4284E+5\r16590.66\t 3.4339E+5\r16584.22\t 3.4439E+5\r16577.79\t 3.4542E+5\r16571.36\t 3.4609E+5\r16564.94\t 3.4634E+5\r16558.53\t 3.4646E+5\r16552.11\t 3.4955E+5\r16545.71\t 3.4942E+5\r16539.30\t 3.5067E+5\r16532.91\t 3.5107E+5\r16526.52\t 3.5193E+5\r16520.13\t 3.5312E+5\r16513.75\t 3.5352E+5\r16507.37\t 3.5452E+5\r16501.00\t 3.5464E+5\r16494.63\t 3.5538E+5\r16488.27\t 3.5638E+5\r16481.91\t 3.5729E+5\r16475.56\t 3.5819E+5\r16469.21\t 3.5893E+5\r16462.87\t 3.5967E+5\r16456.53\t 3.5954E+5\r16450.20\t 3.6083E+5\r16443.87\t 3.6190E+5\r16437.55\t 3.6060E+5\r16431.23\t 3.6248E+5\r16424.92\t 3.6366E+5\r16418.61\t 3.6407E+5\r16412.31\t 3.6474E+5\r16406.01\t 3.6499E+5\r16399.71\t 3.6606E+5\r16393.43\t 3.6693E+5\r16387.14\t 3.6778E+5\r16380.86\t 3.6794E+5\r16374.59\t 3.6864E+5\r16368.32\t 3.6995E+5\r16362.06\t 3.7043E+5\r16355.80\t 3.7132E+5\r16349.54\t 3.7173E+5\r16343.29\t 3.7274E+5\r16337.05\t 3.7340E+5\r16330.81\t 3.7389E+5\r16324.57\t 3.7485E+5\r16318.34\t 3.7464E+5\r16312.12\t 3.7624E+5\r16305.90\t 3.7800E+5\r16299.68\t 3.7786E+5\r16293.47\t 3.7938E+5\r16287.26\t 3.8005E+5\r16281.06\t 3.8063E+5\r16274.86\t 3.8164E+5\r16268.67\t 3.8218E+5\r16262.48\t 3.8223E+5\r16256.30\t 3.8325E+5\r16250.12\t 3.8527E+5\r16243.95\t 3.8538E+5\r16237.78\t 3.8722E+5\r16231.62\t 3.8759E+5\r16225.46\t 3.8798E+5\r16219.30\t 3.8981E+5\r16213.15\t 3.9038E+5\r16207.01\t 3.9103E+5\r16200.87\t 3.9002E+5\r16194.73\t 3.9237E+5\r16188.60\t 3.9361E+5\r16182.48\t 3.9422E+5\r16176.36\t 3.9472E+5\r16170.24\t 3.9577E+5\r16164.13\t 3.9709E+5\r16158.02\t 3.9780E+5\r16151.92\t 3.9848E+5\r16145.82\t 3.9813E+5\r16139.73\t 3.9986E+5\r16133.64\t 4.0087E+5\r16127.55\t 4.0186E+5\r16121.47\t 4.0207E+5\r16115.40\t 4.0302E+5\r16109.33\t 4.0432E+5\r16103.26\t 4.0507E+5\r16097.20\t 4.0621E+5\r16091.14\t 4.0716E+5\r16085.09\t 4.0614E+5\r16079.04\t 4.0892E+5\r16073.00\t 4.1076E+5\r16066.96\t 4.1097E+5\r16060.93\t 4.1226E+5\r16054.90\t 4.1342E+5\r16048.88\t 4.1489E+5\r16042.86\t 4.1580E+5\r16036.84\t 4.1696E+5\r16030.83\t 4.1748E+5\r16024.83\t 4.1797E+5\r16018.82\t 4.2091E+5\r16012.83\t 4.2176E+5\r16006.83\t 4.2245E+5\r16000.85\t 4.2502E+5\r15994.86\t 4.2552E+5\r15988.88\t 4.2733E+5\r15982.91\t 4.2906E+5\r15976.94\t 4.3020E+5\r15970.97\t 4.2979E+5\r15965.01\t 4.3338E+5\r15959.06\t 4.3455E+5\r15953.10\t 4.3580E+5\r15947.16\t 4.3746E+5\r15941.21\t 4.3959E+5\r15935.28\t 4.4120E+5\r15929.34\t 4.4214E+5\r15923.41\t 4.4401E+5\r15917.49\t 4.4408E+5\r15911.57\t 4.4749E+5\r15905.65\t 4.4967E+5\r15899.74\t 4.4993E+5\r15893.83\t 4.5171E+5\r15887.93\t 4.5333E+5\r15882.03\t 4.5434E+5\r15876.14\t 4.5601E+5\r15870.25\t 4.5902E+5\r15864.36\t 4.5917E+5\r15858.48\t 4.5965E+5\r15852.60\t 4.6349E+5\r15846.73\t 4.6492E+5\r15840.86\t 4.6622E+5\r15835.00\t 4.6714E+5\r15829.14\t 4.6979E+5\r15823.29\t 4.7047E+5\r15817.44\t 4.7155E+5\r15811.59\t 4.7346E+5\r15805.75\t 4.7317E+5\r15799.91\t 4.7651E+5\r15794.08\t 4.7813E+5\r15788.25\t 4.7995E+5\r15782.43\t 4.8170E+5\r15776.61\t 4.8261E+5\r15770.79\t 4.8472E+5\r15764.98\t 4.8631E+5\r15759.18\t 4.8736E+5\r15753.37\t 4.8871E+5\r15747.58\t 4.8848E+5\r15741.78\t 4.9153E+5\r15735.99\t 4.9368E+5\r15730.21\t 4.9403E+5\r15724.43\t 4.9633E+5\r15718.65\t 4.9671E+5\r15712.88\t 4.9904E+5\r15707.11\t 5.0066E+5\r15701.35\t 5.0206E+5\r15695.59\t 5.0175E+5\r15689.83\t 5.0512E+5\r15684.08\t 5.0708E+5\r15678.34\t 5.0908E+5\r15672.59\t 5.1041E+5\r15666.86\t 5.1140E+5\r15661.12\t 5.1395E+5\r15655.39\t 5.1583E+5\r15649.67\t 5.1688E+5\r15643.95\t 5.1802E+5\r15638.23\t 5.1788E+5\r15632.52\t 5.2181E+5\r15626.81\t 5.2263E+5\r15621.10\t 5.2404E+5\r15615.40\t 5.2602E+5\r15609.71\t 5.2640E+5\r15604.02\t 5.2765E+5\r15598.33\t 5.2951E+5\r15592.65\t 5.3111E+5\r15586.97\t 5.3010E+5\r15581.29\t 5.3412E+5\r15575.62\t 5.3487E+5\r15569.95\t 5.3682E+5\r15564.29\t 5.3782E+5\r15558.63\t 5.3861E+5\r15552.98\t 5.3978E+5\r15547.33\t 5.4201E+5\r15541.68\t 5.4195E+5\r15536.04\t 5.4399E+5\r15530.40\t 5.4298E+5\r15524.77\t 5.4590E+5\r15519.14\t 5.4633E+5\r15513.52\t 5.4766E+5\r15507.90\t 5.4808E+5\r15502.28\t 5.4981E+5\r15496.67\t 5.5034E+5\r15491.06\t 5.5157E+5\r15485.45\t 5.5333E+5\r15479.85\t 5.5144E+5\r15474.26\t 5.5470E+5\r15468.66\t 5.5568E+5\r15463.08\t 5.5765E+5\r15457.49\t 5.5844E+5\r15451.91\t 5.5922E+5\r15446.34\t 5.5996E+5\r15440.77\t 5.6133E+5\r15435.20\t 5.6240E+5\r15429.63\t 5.6230E+5\r15424.07\t 5.6174E+5\r15418.52\t 5.6455E+5\r15412.97\t 5.6512E+5\r15407.42\t 5.6641E+5\r15401.88\t 5.6654E+5\r15396.34\t 5.6760E+5\r15390.80\t 5.6926E+5\r15385.27\t 5.6937E+5\r15379.74\t 5.7062E+5\r15374.22\t 5.6970E+5\r15368.70\t 5.7311E+5\r15363.18\t 5.7428E+5\r15357.67\t 5.7445E+5\r15352.17\t 5.7522E+5\r15346.66\t 5.7696E+5\r15341.16\t 5.7757E+5\r15335.67\t 5.8010E+5\r15330.18\t 5.8038E+5\r15324.69\t 5.8152E+5\r15319.20\t 5.8138E+5\r15313.73\t 5.8527E+5\r15308.25\t 5.8654E+5\r15302.78\t 5.8726E+5\r15297.31\t 5.8906E+5\r15291.85\t 5.9024E+5\r15286.39\t 5.9150E+5\r15280.93\t 5.9304E+5\r15275.48\t 5.9434E+5\r15270.03\t 5.9342E+5\r15264.59\t 5.9637E+5\r15259.15\t 5.9770E+5\r15253.71\t 5.9857E+5\r15248.28\t 6.0115E+5\r15242.85\t 6.0180E+5\r15237.43\t 6.0491E+5\r15232.01\t 6.0679E+5\r15226.59\t 6.0748E+5\r15221.18\t 6.0814E+5\r15215.77\t 6.0952E+5\r15210.36\t 6.1245E+5\r15204.96\t 6.1367E+5\r15199.57\t 6.1466E+5\r15194.17\t 6.1513E+5\r15188.78\t 6.1633E+5\r15183.40\t 6.1705E+5\r15178.02\t 6.1805E+5\r15172.64\t 6.2039E+5\r15167.26\t 6.2019E+5\r15161.89\t 6.2418E+5\r15156.53\t 6.2554E+5\r15151.16\t 6.2679E+5\r15145.81\t 6.2882E+5\r15140.45\t 6.2900E+5\r15135.10\t 6.3062E+5\r15129.75\t 6.3150E+5\r15124.41\t 6.3266E+5\r15119.07\t 6.3282E+5\r15113.73\t 6.3513E+5\r15108.40\t 6.3765E+5\r15103.07\t 6.3856E+5\r15097.75\t 6.3916E+5\r15092.43\t 6.4043E+5\r15087.11\t 6.4103E+5\r15081.80\t 6.4284E+5\r15076.49\t 6.4402E+5\r15071.19\t 6.4484E+5\r15065.88\t 6.4368E+5\r15060.59\t 6.4682E+5\r15055.29\t 6.4871E+5\r15050.00\t 6.4966E+5\r15044.72\t 6.4944E+5\r15039.43\t 6.5092E+5\r15034.15\t 6.5272E+5\r15028.88\t 6.5345E+5\r15023.61\t 6.5462E+5\r15018.34\t 6.5478E+5\r15013.08\t 6.5643E+5\r15007.82\t 6.5746E+5\r15002.56\t 6.5757E+5\r14997.31\t 6.5932E+5\r14992.06\t 6.5940E+5\r14986.81\t 6.6068E+5\r14981.57\t 6.6177E+5\r14976.33\t 6.6213E+5\r14971.10\t 6.6236E+5\r14965.87\t 6.6108E+5\r14960.64\t 6.6442E+5\r14955.42\t 6.6432E+5\r14950.20\t 6.6530E+5\r14944.98\t 6.6576E+5\r14939.77\t 6.6558E+5\r14934.56\t 6.6622E+5\r14929.36\t 6.6722E+5\r14924.16\t 6.6734E+5\r14918.96\t 6.6626E+5\r14913.76\t 6.6619E+5\r14908.57\t 6.6720E+5\r14903.39\t 6.6677E+5\r14898.21\t 6.6762E+5\r14893.03\t 6.6753E+5\r14887.85\t 6.6711E+5\r14882.68\t 6.6725E+5\r14877.51\t 6.6686E+5\r14872.35\t 6.6659E+5\r14867.19\t 6.6435E+5\r14862.03\t 6.6720E+5\r14856.87\t 6.6688E+5\r14851.72\t 6.6652E+5\r14846.58\t 6.6611E+5\r14841.43\t 6.6508E+5\r14836.30\t 6.6470E+5\r14831.16\t 6.6599E+5\r14826.03\t 6.6464E+5\r14820.90\t 6.6342E+5\r14815.77\t 6.6224E+5\r14810.65\t 6.6281E+5\r14805.54\t 6.6305E+5\r14800.42\t 6.6260E+5\r14795.31\t 6.6203E+5\r14790.20\t 6.6216E+5\r14785.10\t 6.6078E+5\r14780.00\t 6.6013E+5\r14774.90\t 6.5787E+5\r14769.81\t 6.5580E+5\r14764.72\t 6.5822E+5\r14759.64\t 6.5780E+5\r14754.55\t 6.5563E+5\r14749.48\t 6.5412E+5\r14744.40\t 6.5457E+5\r14739.33\t 6.5266E+5\r14734.26\t 6.5206E+5\r14729.20\t 6.5174E+5\r14724.14\t 6.4951E+5\r14719.08\t 6.4785E+5\r14714.02\t 6.4732E+5\r14708.97\t 6.4601E+5\r14703.93\t 6.4461E+5\r14698.88\t 6.4242E+5\r14693.84\t 6.4022E+5\r14688.81\t 6.4034E+5\r14683.78\t 6.3899E+5\r14678.75\t 6.3710E+5\r14673.72\t 6.3382E+5\r14668.70\t 6.3432E+5\r14663.68\t 6.3292E+5\r14658.66\t 6.3198E+5\r14653.65\t 6.3080E+5\r14648.64\t 6.2909E+5\r14643.64\t 6.2885E+5\r14638.64\t 6.2716E+5\r14633.64\t 6.2559E+5\r14628.64\t 6.2313E+5\r14623.65\t 6.2144E+5\r14618.66\t 6.2155E+5\r14613.68\t 6.2070E+5\r14608.70\t 6.1850E+5\r14603.72\t 6.1788E+5\r14598.75\t 6.1622E+5\r14593.78\t 6.1547E+5\r14588.81\t 6.1263E+5\r14583.85\t 6.1117E+5\r14578.89\t 6.0743E+5\r14573.93\t 6.0860E+5\r14568.98\t 6.0689E+5\r14564.03\t 6.0442E+5\r14559.08\t 6.0327E+5\r14554.14\t 6.0159E+5\r14549.20\t 5.9946E+5\r14544.26\t 5.9745E+5\r14539.33\t 5.9609E+5\r14534.40\t 5.9265E+5\r14529.47\t 5.9176E+5\r14524.55\t 5.9109E+5\r14519.63\t 5.8922E+5\r14514.71\t 5.8632E+5\r14509.80\t 5.8606E+5\r14504.89\t 5.8404E+5\r14499.98\t 5.8141E+5\r14495.08\t 5.8085E+5\r14490.18\t 5.7845E+5\r14485.29\t 5.7431E+5\r14480.39\t 5.7476E+5\r14475.50\t 5.7294E+5\r14470.62\t 5.7098E+5\r14465.74\t 5.6959E+5\r14460.86\t 5.6781E+5\r14455.98\t 5.6560E+5\r14451.11\t 5.6376E+5\r14446.24\t 5.6190E+5\r14441.37\t 5.5760E+5\r14436.51\t 5.5722E+5\r14431.65\t 5.5464E+5\r14426.79\t 5.5240E+5\r14421.94\t 5.5148E+5\r14417.09\t 5.4970E+5\r14412.25\t 5.4805E+5\r14407.40\t 5.4689E+5\r14402.56\t 5.4514E+5\r14397.73\t 5.4251E+5\r14392.89\t 5.3800E+5\r14388.07\t 5.3808E+5\r14383.24\t 5.3677E+5\r14378.42\t 5.3401E+5\r14373.60\t 5.3183E+5\r14368.78\t 5.3064E+5\r14363.97\t 5.2932E+5\r14359.16\t 5.2724E+5\r14354.35\t 5.2500E+5\r14349.55\t 5.2096E+5\r14344.75\t 5.2107E+5\r14339.95\t 5.2017E+5\r14335.16\t 5.1821E+5\r14330.36\t 5.1621E+5\r14325.58\t 5.1502E+5\r14320.79\t 5.1295E+5\r14316.01\t 5.1172E+5\r14311.24\t 5.1062E+5\r14306.46\t 5.0839E+5\r14301.69\t 5.0395E+5\r14296.92\t 5.0451E+5\r14292.16\t 5.0357E+5\r14287.40\t 5.0127E+5\r14282.64\t 5.0023E+5\r14277.88\t 4.9829E+5\r14273.13\t 4.9732E+5\r14268.38\t 4.9681E+5\r14263.64\t 4.9393E+5\r14258.90\t 4.9082E+5\r14254.16\t 4.9156E+5\r14249.42\t 4.8996E+5\r14244.69\t 4.8931E+5\r14239.96\t 4.8682E+5\r14235.23\t 4.8520E+5\r14230.51\t 4.8436E+5\r14225.79\t 4.8168E+5\r14221.07\t 4.8035E+5\r14216.36\t 4.7860E+5\r14211.65\t 4.7480E+5\r14206.94\t 4.7477E+5\r14202.24\t 4.7246E+5\r14197.54\t 4.7152E+5\r14192.84\t 4.6930E+5\r14188.14\t 4.6732E+5\r14183.45\t 4.6524E+5\r14178.76\t 4.6343E+5\r14174.08\t 4.6163E+5\r14169.40\t 4.5697E+5\r14164.72\t 4.5757E+5\r14160.04\t 4.5566E+5\r14155.37\t 4.5312E+5\r14150.70\t 4.5093E+5\r14146.03\t 4.4898E+5\r14141.37\t 4.4619E+5\r14136.71\t 4.4485E+5\r14132.05\t 4.4335E+5\r14127.40\t 4.4104E+5\r14122.75\t 4.3688E+5\r14118.10\t 4.3614E+5\r14113.46\t 4.3442E+5\r14108.82\t 4.3233E+5\r14104.18\t 4.3031E+5\r14099.54\t 4.2848E+5\r14094.91\t 4.2604E+5\r14090.28\t 4.2490E+5\r14085.65\t 4.2261E+5\r14081.03\t 4.1938E+5\r14076.41\t 4.1843E+5\r14071.79\t 4.1663E+5\r14067.18\t 4.1629E+5\r14062.57\t 4.1430E+5\r14057.96\t 4.1250E+5\r14053.36\t 4.1140E+5\r14048.76\t 4.1006E+5\r14044.16\t 4.0866E+5\r14039.56\t 4.0707E+5\r14034.97\t 4.0329E+5\r14030.38\t 4.0309E+5\r14025.79\t 4.0190E+5\r14021.21\t 4.0024E+5\r14016.63\t 3.9905E+5\r14012.05\t 3.9745E+5\r14007.48\t 3.9558E+5\r14002.91\t 3.9444E+5\r13998.34\t 3.9371E+5\r13993.78\t 3.9026E+5\r13989.21\t 3.9064E+5\r13984.65\t 3.8828E+5\r13980.10\t 3.8653E+5\r13975.55\t 3.8564E+5\r13971.00\t 3.8444E+5\r13966.45\t 3.8257E+5\r13961.90\t 3.8180E+5\r13957.36\t 3.8100E+5\r13952.83\t 3.7872E+5\r13948.29\t 3.7739E+5\r13943.76\t 3.7685E+5\r13939.23\t 3.7520E+5\r13934.70\t 3.7432E+5\r13930.18\t 3.7310E+5\r13925.66\t 3.7122E+5\r13921.14\t 3.7001E+5\r13916.63\t 3.6887E+5\r13912.12\t 3.6756E+5\r13907.61\t 3.6468E+5\r13903.10\t 3.6451E+5\r13898.60\t 3.6313E+5\r13894.10\t 3.6130E+5\r13889.61\t 3.6006E+5\r13885.11\t 3.5874E+5\r13880.62\t 3.5736E+5\r13876.13\t 3.5599E+5\r13871.65\t 3.5473E+5\r13867.17\t 3.5287E+5\r13862.69\t 3.5167E+5\r13858.21\t 3.5157E+5\r13853.74\t 3.5056E+5\r13849.27\t 3.4943E+5\r13844.80\t 3.4928E+5\r13840.34\t 3.4811E+5\r13835.88\t 3.4881E+5\r13831.42\t 3.4824E+5\r13826.97\t 3.4784E+5\r13822.51\t 3.4610E+5\r13818.06\t 3.4760E+5\r13813.62\t 3.4765E+5\r13809.17\t 3.4834E+5\r13804.73\t 3.4853E+5\r13800.29\t 3.4879E+5\r13795.86\t 3.4890E+5\r13791.43\t 3.4849E+5\r13787.00\t 3.4923E+5\r13782.57\t 3.4862E+5\r13778.15\t 3.4772E+5\r13773.73\t 3.4904E+5\r13769.31\t 3.4882E+5\r13764.89\t 3.4816E+5\r13760.48\t 3.4837E+5\r13756.07\t 3.4881E+5\r13751.67\t 3.4841E+5\r13747.26\t 3.4844E+5\r13742.86\t 3.4809E+5\r13738.47\t 3.4644E+5\r13734.07\t 3.4753E+5\r13729.68\t 3.4751E+5\r13725.29\t 3.4719E+5\r13720.90\t 3.4698E+5\r13716.52\t 3.4697E+5\r13712.14\t 3.4738E+5\r13707.76\t 3.4665E+5\r13703.39\t 3.4666E+5\r13699.02\t 3.4616E+5\r13694.65\t 3.4554E+5\r13690.28\t 3.4611E+5\r13685.92\t 3.4625E+5\r13681.56\t 3.4610E+5\r13677.20\t 3.4613E+5\r13672.84\t 3.4536E+5\r13668.49\t 3.4587E+5\r13664.14\t 3.4610E+5\r13659.79\t 3.4555E+5\r13655.45\t 3.4444E+5\r13651.11\t 3.4553E+5\r13646.77\t 3.4528E+5\r13642.43\t 3.4573E+5\r13638.10\t 3.4562E+5\r13633.77\t 3.4501E+5\r13629.44\t 3.4501E+5\r13625.12\t 3.4517E+5\r13620.80\t 3.4532E+5\r13616.48\t 3.4374E+5\r13612.16\t 3.4422E+5\r13607.85\t 3.4506E+5\r13603.54\t 3.4433E+5\r13599.23\t 3.4513E+5\r13594.93\t 3.4478E+5\r13590.63\t 3.4476E+5\r13586.33\t 3.4458E+5\r13582.03\t 3.4490E+5\r13577.74\t 3.4456E+5\r13573.45\t 3.4302E+5\r13569.16\t 3.4362E+5\r13564.87\t 3.4359E+5\r13560.59\t 3.4378E+5\r13556.31\t 3.4291E+5\r13552.03\t 3.4350E+5\r13547.76\t 3.4313E+5\r13543.48\t 3.4392E+5\r13539.22\t 3.4312E+5\r13534.95\t 3.4265E+5\r13530.69\t 3.4261E+5\r13526.42\t 3.4304E+5\r13522.17\t 3.4304E+5\r13517.91\t 3.4278E+5\r13513.66\t 3.4274E+5\r13509.41\t 3.4216E+5\r13505.16\t 3.4175E+5\r13500.92\t 3.4121E+5\r13496.67\t 3.4092E+5\r13492.43\t 3.3902E+5\r13488.20\t 3.4038E+5\r13483.96\t 3.3905E+5\r13479.73\t 3.3835E+5\r13475.50\t 3.3757E+5\r13471.28\t 3.3710E+5\r13467.06\t 3.3635E+5\r13462.83\t 3.3580E+5\r13458.62\t 3.3551E+5\r13454.40\t 3.3394E+5\r13450.19\t 3.3338E+5\r13445.98\t 3.3412E+5\r13441.77\t 3.3405E+5\r13437.57\t 3.3363E+5\r13433.37\t 3.3451E+5\r13429.17\t 3.3490E+5\r13424.97\t 3.3570E+5\r13420.78\t 3.3726E+5\r13416.59\t 3.3881E+5\r13412.40\t 3.3909E+5\r13408.21\t 3.4302E+5\r13404.03\t 3.4565E+5\r13399.85\t 3.4753E+5\r13395.67\t 3.5099E+5\r13391.50\t 3.5405E+5\r13387.32\t 3.5738E+5\r13383.15\t 3.6065E+5\r13378.99\t 3.6390E+5\r13374.82\t 3.6558E+5\r13370.66\t 3.6954E+5\r13366.50\t 3.7347E+5\r13362.35\t 3.7525E+5\r13358.19\t 3.7775E+5\r13354.04\t 3.7981E+5\r13349.89\t 3.8175E+5\r13345.74\t 3.8341E+5\r13341.60\t 3.8450E+5\r13337.46\t 3.8660E+5\r13333.32\t 3.8560E+5\r13329.19\t 3.8793E+5\r13325.05\t 3.8991E+5\r13320.92\t 3.9052E+5\r13316.79\t 3.9170E+5\r13312.67\t 3.9205E+5\r13308.55\t 3.9196E+5\r13304.43\t 3.9173E+5\r13300.31\t 3.9245E+5\r13296.19\t 3.9069E+5\r13292.08\t 3.9305E+5\r13287.97\t 3.9285E+5\r13283.86\t 3.9358E+5\r13279.76\t 3.9408E+5\r13275.66\t 3.9282E+5\r13271.56\t 3.9318E+5\r13267.46\t 3.9287E+5\r13263.37\t 3.9297E+5\r13259.28\t 3.9326E+5\r13255.19\t 3.9086E+5\r13251.10\t 3.9151E+5\r13247.02\t 3.9133E+5\r13242.93\t 3.9043E+5\r13238.86\t 3.8930E+5\r13234.78\t 3.8892E+5\r13230.71\t 3.8867E+5\r13226.63\t 3.8815E+5\r13222.57\t 3.8810E+5\r13218.50\t 3.8696E+5\r13214.44\t 3.8804E+5\r13210.37\t 3.8865E+5\r13206.32\t 3.8773E+5\r13202.26\t 3.8797E+5\r13198.21\t 3.8688E+5\r13194.15\t 3.8700E+5\r13190.11\t 3.8642E+5\r13186.06\t 3.8699E+5\r13182.02\t 3.8591E+5\r13177.98\t 3.8351E+5\r13173.94\t 3.8478E+5\r13169.90\t 3.8403E+5\r13165.87\t 3.8408E+5\r13161.84\t 3.8318E+5\r13157.81\t 3.8183E+5\r13153.78\t 3.8158E+5\r13149.76\t 3.8141E+5\r13145.74\t 3.8192E+5\r13141.72\t 3.7982E+5\r13137.70\t 3.8140E+5\r13133.69\t 3.8126E+5\r13129.68\t 3.8148E+5\r13125.67\t 3.8122E+5\r13121.67\t 3.8116E+5\r13117.66\t 3.8022E+5\r13113.66\t 3.7949E+5\r13109.66\t 3.7953E+5\r13105.67\t 3.7914E+5\r13101.67\t 3.7753E+5\r13097.68\t 3.7827E+5\r13093.69\t 3.7783E+5\r13089.71\t 3.7761E+5\r13085.72\t 3.7694E+5\r13081.74\t 3.7651E+5\r13077.76\t 3.7608E+5\r13073.79\t 3.7589E+5\r13069.81\t 3.7623E+5\r13065.84\t 3.7367E+5\r13061.87\t 3.7480E+5\r13057.91\t 3.7429E+5\r13053.94\t 3.7396E+5\r13049.98\t 3.7311E+5\r13046.02\t 3.7333E+5\r13042.07\t 3.7276E+5\r13038.11\t 3.7168E+5\r13034.16\t 3.7186E+5\r13030.21\t 3.7130E+5\r13026.26\t 3.6785E+5\r13022.32\t 3.6894E+5\r13018.38\t 3.6829E+5\r13014.44\t 3.6774E+5\r13010.50\t 3.6763E+5\r13006.57\t 3.6649E+5\r13002.63\t 3.6659E+5\r12998.70\t 3.6540E+5\r12994.78\t 3.6470E+5\r12990.85\t 3.6236E+5\r12986.93\t 3.6278E+5\r12983.01\t 3.6246E+5\r12979.09\t 3.6160E+5\r12975.17\t 3.6141E+5\r12971.26\t 3.6071E+5\r12967.35\t 3.5993E+5\r12963.44\t 3.5922E+5\r12959.54\t 3.5809E+5\r12955.63\t 3.5803E+5\r12951.73\t 3.5568E+5\r12947.83\t 3.5697E+5\r12943.94\t 3.5570E+5\r12940.04\t 3.5597E+5\r12936.15\t 3.5513E+5\r12932.26\t 3.5498E+5\r12928.38\t 3.5447E+5\r12924.49\t 3.5412E+5\r12920.61\t 3.5361E+5\r12916.73\t 3.5192E+5\r12912.85\t 3.5343E+5\r12908.98\t 3.5373E+5\r12905.10\t 3.5324E+5\r12901.23\t 3.5281E+5\r12897.37\t 3.5273E+5\r12893.50\t 3.5293E+5\r12889.64\t 3.5323E+5\r12885.78\t 3.5299E+5\r12881.92\t 3.5232E+5\r12878.06\t 3.5237E+5\r12874.21\t 3.5310E+5\r12870.36\t 3.5353E+5\r12866.51\t 3.5411E+5\r12862.66\t 3.5331E+5\r12858.82\t 3.5472E+5\r12854.97\t 3.5482E+5\r12851.13\t 3.5509E+5\r12847.30\t 3.5600E+5\r12843.46\t 3.5473E+5\r12839.63\t 3.5676E+5\r12835.80\t 3.5756E+5\r12831.97\t 3.5807E+5\r12828.15\t 3.5837E+5\r12824.32\t 3.5930E+5\r12820.50\t 3.5998E+5\r12816.68\t 3.6114E+5\r12812.87\t 3.6224E+5\r12809.05\t 3.6230E+5\r12805.24\t 3.6285E+5\r12801.43\t 3.6422E+5\r12797.62\t 3.6553E+5\r12793.82\t 3.6674E+5\r12790.01\t 3.6740E+5\r12786.21\t 3.6879E+5\r12782.42\t 3.6932E+5\r12778.62\t 3.7069E+5\r12774.83\t 3.7224E+5\r12771.04\t 3.7066E+5\r12767.25\t 3.7408E+5\r12763.46\t 3.7497E+5\r12759.68\t 3.7600E+5\r12755.89\t 3.7727E+5\r12752.11\t 3.7852E+5\r12748.34\t 3.7988E+5\r12744.56\t 3.8166E+5\r12740.79\t 3.8319E+5\r12737.02\t 3.8407E+5\r12733.25\t 3.8414E+5\r12729.48\t 3.8626E+5\r12725.72\t 3.8828E+5\r12721.96\t 3.8960E+5\r12718.20\t 3.9117E+5\r12714.44\t 3.9292E+5\r12710.69\t 3.9380E+5\r12706.93\t 3.9568E+5\r12703.18\t 3.9707E+5\r12699.44\t 3.9712E+5\r12695.69\t 4.0047E+5\r12691.95\t 4.0173E+5\r12688.21\t 4.0379E+5\r12684.47\t 4.0606E+5\r12680.73\t 4.0691E+5\r12676.99\t 4.0863E+5\r12673.26\t 4.1108E+5\r12669.53\t 4.1356E+5\r12665.80\t 4.1308E+5\r12662.08\t 4.1562E+5\r12658.36\t 4.1827E+5\r12654.63\t 4.1942E+5\r12650.92\t 4.2162E+5\r12647.20\t 4.2398E+5\r12643.48\t 4.2618E+5\r12639.77\t 4.2790E+5\r12636.06\t 4.2993E+5\r12632.35\t 4.3109E+5\r12628.65\t 4.3204E+5\r12624.94\t 4.3534E+5\r12621.24\t 4.3700E+5\r12617.54\t 4.3923E+5\r12613.85\t 4.4118E+5\r12610.15\t 4.4282E+5\r12606.46\t 4.4516E+5\r12602.77\t 4.4741E+5\r12599.08\t 4.4881E+5\r12595.40\t 4.5042E+5\r12591.71\t 4.5210E+5\r12588.03\t 4.5396E+5\r12584.35\t 4.5659E+5\r12580.68\t 4.5736E+5\r12577.00\t 4.6020E+5\r12573.33\t 4.6221E+5\r12569.66\t 4.6429E+5\r12565.99\t 4.6605E+5\r12562.32\t 4.6730E+5\r12558.66\t 4.6704E+5\r12555.00\t 4.7087E+5\r12551.34\t 4.7249E+5\r12547.68\t 4.7502E+5\r12544.02\t 4.7660E+5\r12540.37\t 4.7985E+5\r12536.72\t 4.8177E+5\r12533.07\t 4.8383E+5\r12529.43\t 4.8577E+5\r12525.78\t 4.8724E+5\r12522.14\t 4.8949E+5\r12518.50\t 4.9169E+5\r12514.86\t 4.9303E+5\r12511.22\t 4.9582E+5\r12507.59\t 4.9776E+5\r12503.96\t 4.9975E+5\r12500.33\t 5.0215E+5\r12496.70\t 5.0460E+5\r12493.08\t 5.0783E+5\r12489.45\t 5.0569E+5\r12485.83\t 5.1010E+5\r12482.22\t 5.1233E+5\r12478.60\t 5.1474E+5\r12474.98\t 5.1642E+5\r12471.37\t 5.1799E+5\r12467.76\t 5.2002E+5\r12464.15\t 5.2163E+5\r12460.55\t 5.2358E+5\r12456.94\t 5.2416E+5\r12453.34\t 5.2529E+5\r12449.74\t 5.2861E+5\r12446.15\t 5.2924E+5\r12442.55\t 5.3182E+5\r12438.96\t 5.3372E+5\r12435.37\t 5.3657E+5\r12431.78\t 5.3764E+5\r12428.19\t 5.3953E+5\r12424.61\t 5.4101E+5\r12421.02\t 5.4203E+5\r12417.44\t 5.4508E+5\r12413.86\t 5.4704E+5\r12410.29\t 5.4883E+5\r12406.71\t 5.5091E+5\r12403.14\t 5.5194E+5\r12399.57\t 5.5373E+5\r12396.00\t 5.5610E+5\r12392.44\t 5.5678E+5\r12388.87\t 5.5754E+5\r12385.31\t 5.6036E+5\r12381.75\t 5.6249E+5\r12378.19\t 5.6342E+5\r12374.64\t 5.6589E+5\r12371.09\t 5.6584E+5\r12367.53\t 5.5684E+5\r"
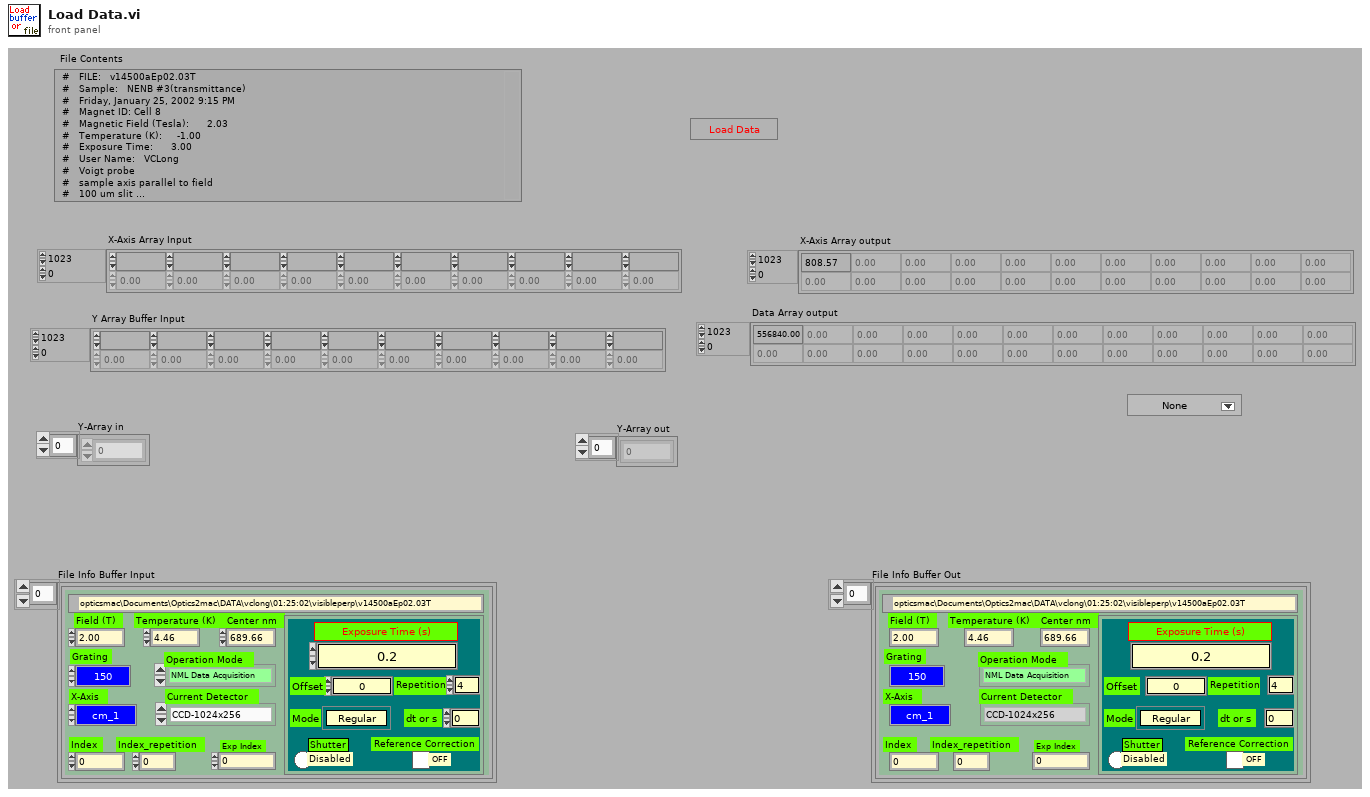
[diagram p1: front panel]
types:
  T1 = typedef "FileInfoParameter.ctt" = cluster{"FilePath":path, "Field (T)":dbl, "Temperature (K)":dbl, "X-Axis":T2, "Center nm":dbl, "Current Grating Density":T3, "CCD Parameters":T4, "Operation Mode":T5, "Exp Index":u32, "Index_repetition":u16, "Index":u16, "Current Detector":T6}
  T2 = typedef "Wavelength Unit.ctt" = enum8{"Point", "nm", "eV", "meV", "cm_1"}
  T3 = typedef "McPherson Grating Density.ctl" = enum8{"150", "300", "600", "1200", "1800"}
  T4 = typedef "CCDParameter.ctt" = cluster{"Exposure Time (s)":dbl, "Offset":dbl, "BkgrdCrct":bool, "Shutter":bool, "Mode":enum8{"Regular", "OverExp Cor", "SpikeRemove", "ForCalibration"}, "Repetition":u16, "dt or s":dbl}
  T5 = typedef "OperationMode.ctt" = enum16{"Standby", "CCD Single Shot", "CCD Sequence Shots", "CCD Custom Shots", "CCD Reference Shot", "Step Scanning ", "Time Scanning", "NML Data Acquisition"}
  T6 = typedef "ListOfDetectors.ctt" = enum8{"CCD-1024x256", "InGaAs PDA-1024x1", "CCD-1340x400", "Ge Single Channel", "Si Single Channel", "PMT Single Channel"}
  T7 = typedef "3 way Status.ctl" = u8
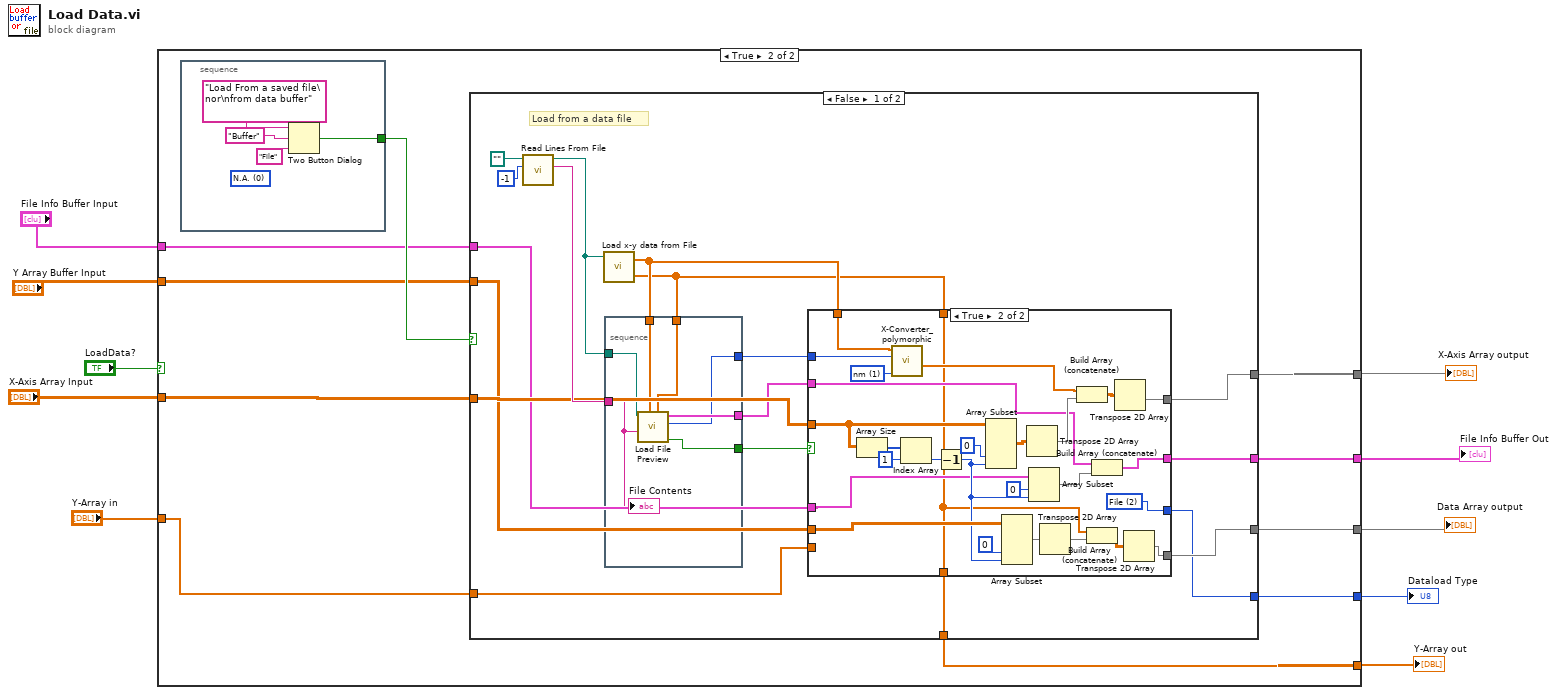
[diagram p0: block diagram]
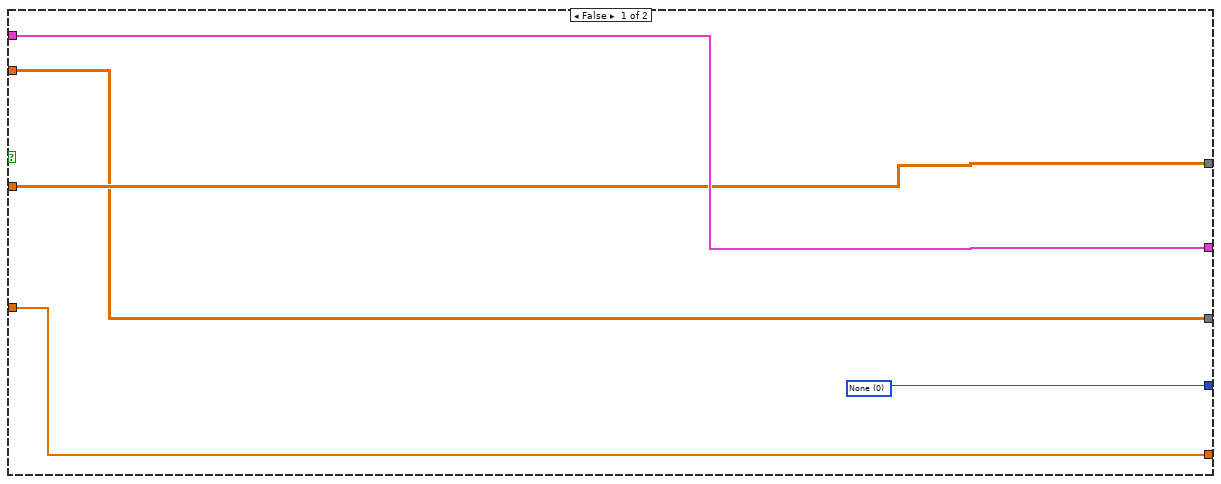
[diagram p2: hidden frame]
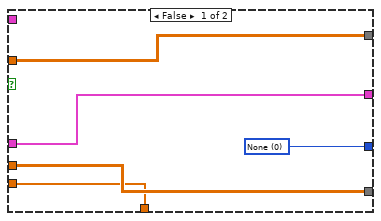
[diagram p3: hidden frame]
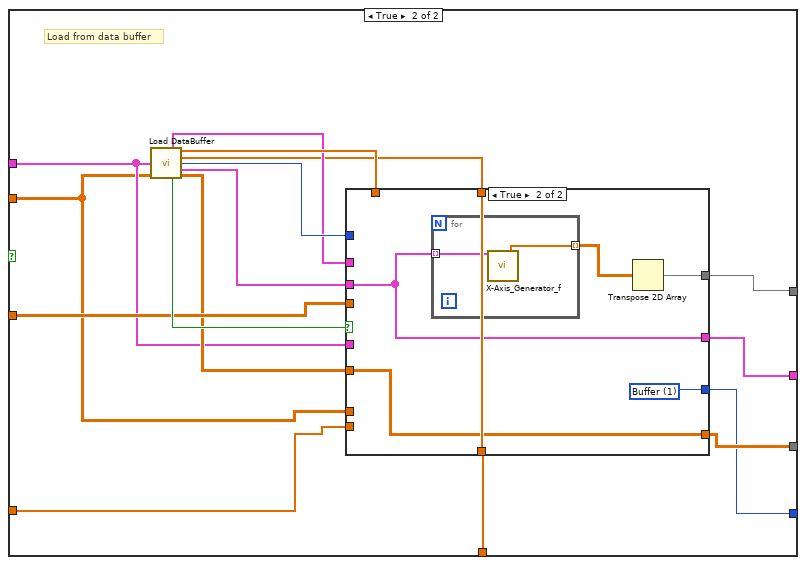
[diagram p4: hidden frame]
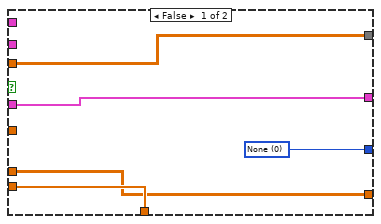
[diagram p5: hidden frame]
diagram:
  n1 = case shown="True" "LoadData?" {
    tunnel: "File Info Buffer Input" -> [w15 w24]
    tunnel: "Y Array Buffer Input" -> [w13 w23]
    tunnel: [w15 w22] -> w8
    tunnel: [w14 w21] -> w7
    tunnel: [w13 w20] -> w6
    tunnel: "X-Axis Array Input" -> [w14 w19]
    tunnel: [w12 w18] -> w4
    tunnel: [w11 w17] -> w3
    tunnel: "Y-Array in" -> [w11 w16]
    frame False {
      w12 = u8 0 items=["None", "Buffer", "File"] ("Dataload Type")
    }
    frame True {
      n2 = stacked-sequence {
        tunnel: [w29] -> w25
        frame #0 {
          (unwired) T7 0 items=["N.A.", "OK", "Busy", "Done"] ("Buffer")
          n3 = Two Button Dialog(message="Load From a saved file\nor\nfrom data buffer", 1:"File" ("F button name (\"Cancel\")"), 2:"Buffer" ("T button name (\"OK\")")) -> (T button?=w29:bool)
        }
      }
      n4 = case shown="False" w25 {
        tunnel: w24 -> [w39 w88]
        tunnel: w23 -> [w40 w87]
        tunnel: [w43 w94] -> w20
        tunnel: [w38 w96] -> w22
        tunnel: [w41 w95] -> w21
        tunnel: w19 -> [w42 w98]
        tunnel: [w35 w93] -> w18
        tunnel: [w34 w89] -> w17
        tunnel: w16 -> [w33 w90]
        frame False {
          # "Load from a data file"
          n5 = call <vilib>:"Read Lines From File.vi"("file path (dialog if empty)"=path "", "number of lines (all:-1)"=-1) -> ("new file path (Not A Path if cancelled)"=w32:path, "line string"=w45:string)  [unwired: 4 in, 2 out]
          n6 = call "Load x-y data from File.vi"("file path"=w32) -> ("Y-Array"=w30:sgl[], "X-Array"=w31:sgl[])  [unwired: 2 in]
          n7 = stacked-sequence {
            tunnel: w45 -> [w86]
            tunnel: [w85] -> w44
            tunnel: w32 -> [w84]
            tunnel: w31 -> [w83]
            tunnel: w30 -> [w82]
            tunnel: [w81] -> w36
            tunnel: [w80] -> w37
            frame #0 {
              n8 = call "Load File Preview.vi"("Y-Array"=w82, "X-Array"=w83, "File Contents"=w86, "File Path"=w84) -> ("Continue?"=w85:bool, "WL unit copy"=w80:i32, "File Parameter Out"=w81:T1)  [unwired: 3 in]
              "File Contents" <- w86
            }
          }
          n9 = case shown="True" w44 {
            tunnel: [w52 w67] -> w41
            tunnel: [w51 w55] -> w38
            tunnel: [w50 w61] -> w43
            tunnel: w42 -> [w52 w73]
            tunnel: w39 -> [w51 w59]
            tunnel: w40 -> [w50 w62]
            tunnel: w31 -> [_ w79]
            tunnel: w37 -> [_ w77]
            tunnel: w30 -> [_ w53]
            tunnel: w36 -> [_ w56]
            tunnel: [w49 w54] -> w35
            tunnel: [w48 w53] -> w34
            tunnel: w33 -> [w48 _]
            frame False {
              w49 = u8 0 items=["None", "Buffer", "File"] ("Dataload Type")
            }
            frame True {
              w54 = u8 2 items=["None", "Buffer", "File"] ("Dataload Type")
              w78 = 1 items=["Point #", "nm", "eV", "meV", "cm-1"] ("X-Axis Unit")
              n10 = Array Size(array=w73) -> (size(s)=w76:i32[])
              n11 = call-poly "X-Converter_polymorphic.vi"("X-Axis Unit"=w78, "Old X-Axis Unit"=w77, "X-Axis input"=w79) -> ("X-Axis Output"=w69:dbl[])  [unwired: 2 in, 3 out]
              n12 = Index Array(array=w76, index=1) -> (element=w74:i32)
              n13 = Decrement(x=w74) -> (x-1=w60:i32)
              n14 = Array Subset(array=w73, index (col)=0 ("index"), length (col)=w60) -> (w71:dbl[][])  [unwired: 2 in]
              n15 = Array Subset(array=w62, index (col)=0 ("index"), length (col)=w60) -> (w65:dbl[][])  [unwired: 2 in]
              n16 = Transpose 2D Array(2D array=w71) -> (transposed array=w70:dbl[][])
              n17 = Array Subset(array=w59, index=0, length=w60) -> (w57:T1[])
              n18 = Transpose 2D Array(2D array=w65) -> (transposed array=w64:dbl[][])
              n19 = Build Array (concatenate)(w69, w70) -> (w68:dbl[][])
              n20 = Build Array (concatenate)(w53, w64) -> (w63:dbl[][])
              n21 = Build Array (concatenate)(w56, w57) -> (w55:T1[])
              n22 = Transpose 2D Array(2D array=w68) -> (transposed array=w67:dbl[][])
              n23 = Transpose 2D Array(2D array=w63) -> (transposed array=w61:dbl[][])
            }
          }
        }
        frame True {
          # "Load from data buffer"
          n24 = call "Load DataBuffer.vi"("File Info Buffer Init"=w88, "Y Array Buffer Init"=w87) -> ("File Info Out"=w99:T1, "X-Data out"=w101:dbl[], "Y-Data out"=w91:dbl[], "X-Axis"=w100:i32, "File Info Buffer Out"=w92:T1[], "Continue?"=w102:bool, "Y Array Buffer Out"=w97:dbl[][])  [unwired: 7 in]
          n25 = case shown="True" w102 {
            tunnel: [w107 w109] -> w95
            tunnel: [w104 w110] -> w96
            tunnel: [w103 w111] -> w94
            tunnel: w98 -> [w107 _]
            tunnel: w92 -> [_ w110]
            tunnel: w97 -> [_ w111]
            tunnel: w101 -> [_ _]
            tunnel: w100 -> [_ _]
            tunnel: w91 -> [_ w112]
            tunnel: w99 -> [_ _]
            tunnel: [w106 w113] -> w93
            tunnel: [w105 w112] -> w89
            tunnel: w90 -> [w105 _]
            tunnel: w88 -> [w104 _]
            tunnel: w87 -> [w103 _]
            frame False {
              w106 = u8 0 items=["None", "Buffer", "File"] ("Dataload Type")
            }
            frame True {
              w113 = u8 1 items=["None", "Buffer", "File"] ("Dataload Type")
              n26 = for {
                tunnel: w110 -> [w115] mode=indexing
                tunnel: [w114] -> w108 mode=indexing
                n27 = call-poly "X-Axis_Generator_f.vi"("File Info In"=w115) -> ("X-axis  (nm)"=w114:dbl[])  [unwired: 11 in, 7 out]
              }
              n28 = Transpose 2D Array(2D array=w108) -> (transposed array=w109:dbl[][])
            }
          }
        }
      }
    }
  }
  "Data Array output" <- w6
  "X-Axis Array output" <- w7
  "File Info Buffer Out" <- w8
  "Dataload Type" <- w4
  "Y-Array out" <- w3
